vi "HOST_ABEL_Kalman.vi"() -> ()   [LabVIEW 2011]
uses:
  <vilib>/FPGAPlugInAG/PCIe-7852R/niLvFpga_Open_PCIe-7852R.vi
  <vilib>/rvi/interface/common/dynamic/niFpgaDynamicAddResources.vi
  <vilib>/Utility/error.llb/Error Cluster From Error Code.vi
  <vilib>/FPGAPlugInAG/Dynamic/niLvFpga_Run_Dynamic.vi
  <vilib>/RVI Host/nirviSupport.llb/nirviErrorClusterFromErrorCode.vi
  <vilib>/rvi/errors/niLvFpgaAdjustHostInterfaceError.vi
  <vilib>/FPGAPlugInAG/Dynamic/niLvFpga_Reset_Dynamic.vi
  <vilib>/FPGAPlugInAG/Dynamic/niLvFpga_Close_Dynamic.vi
  <vilib>/rvi/interface/nirviOpenFPGA/nirviOpenFPGA.xnode
  FPGA Bitfiles/ABELKalman_FPGATarget_FPGAABELKalman_65AD47D3.lvbitx
  FPGA_ABEL_Kalman.vi
  <vilib>/rvi/interface/nirviMethod/nirviMethod.xnode
  <vilib>/rvi/interface/nirviCloseFPGA/nirviCloseFPGA.xnode
  <vilib>/Analysis/NI_AALBase.lvlib
  <vilib>/rvi/errors/niLvFpgaMergeErrorWithErrorCode.vi
  <vilib>/FPGAPlugInAG/Dynamic/niLvFpga_ConfigureFifo_Dynamic.vi
  <vilib>/FPGAPlugInAG/Dynamic/niLvFpga_StartFifo_Dynamic.vi
  <vilib>/FPGAPlugInAG/Dynamic/niLvFpga_ReadFifo_Dynamic.vi
  <vilib>/FPGAPlugInAG/Dynamic/niLvFpga_WriteFifo_Dynamic.vi
  <vilib>/rvi/interface/nirviMethod/StockFPGA_InlinedMethodWaitForMultipleIRQ.vi
  <vilib>/FPGAPlugInAG/Dynamic/niLvFpga_WaitOnIrq_Dynamic.vi
  <vilib>/FPGAPlugInAG/Dynamic/niLvFpga_AcknowledgeIrq_Dynamic.vi
panel:
  out "Currently Trapped":bool
  out "Number of Trapping Events":u16
  out "Average Time Trapped (ms)":dbl
  in  "Estimate Trap Time":bool
  in  "Threshold (Hz)":dbl=12000.0 min=0.0
  out "Time Recorded (s)":dbl
  in  "Time to Record (s)":dbl=-1.0
  out "Current Modulation Voltages":dbl[][](array[numeric])
  in  "Clear Warnings":bool
  out "y Estimate":dbl
  out "x Estimate":dbl
  in  "Tab Control":enum32{"ABEL Trap Settings"}(tab)
  in  "New Maximum Feedback (V)":dbl=10.0 min=0.0 max=10.0
  out "Current Number of Points per Scan":u8=1
  in  "New Number of Points per Scan":u8=27 min=3 max=32
  in  "New Scan Form":enum8{"Circular", "Square", "Hexagonal"}(ring)=enum."Hexagonal"
  in  "New Spacing (um)":dbl=0.75 min=0.0
  out "Current Scan Form":enum8{"Circular", "Square", "Hexagonal"}(ring)
  out "Current Spacing (um)":dbl
  in  "New Scan Frequency (Hz)":dbl
  out "Current Scan Frequency (Hz)":dbl
  in  "New Radius (um)":dbl min=0.0
  out "Current Radius (um)":dbl
  in  "New Sub-Bin Delay":u16=112
  out "Current Sub-Bin Delay":u16=112
  in  "New Diffusion Constant Estimate (um^2/s)":dbl min=0.0
  out "Current Diffusion Constant Estimate (um^2/s)":dbl
  in  "New Mobility Estimate (um/s/V)":dbl
  out "Current Mobility Estimate (um/s/V)":dbl
  in  "New Beam Waist Estimate (um)":dbl=0.36 min=0.0
  out "Current Beam Waist Estimate (um)":dbl
  in  "New EOD Deflection Scale (um/V)":dbl=0.21 min=0.0
  out "Current EOD Deflection Scale (um/V)":dbl
  out "Current Maximum Feedback (V)":dbl
  out "Current Modulation Frequency (Hz)":dbl
  in  "New Modulation Frequency (Hz)":dbl min=0.0
  out "Current Modulation Radius (um)":dbl
  in  "New Modulation Radius (um)":dbl min=0.0
  in  "New Number of Modulation Points":u8=1 min=1 max=16
  out "Current Number of Modulation Points":u8=1
  in  "New Modulation Angle (degrees)":dbl min=0.0 max=360.0
  out "Current Modulation Angle (degrees)":dbl
  out "On-Chip FIFO Overflow":bool
  in  "Include Mobility Update":bool
  in  "Trap":bool
  out "Feedback DMA Overflow":bool
  out "Feedback":dbl(slide) scale=0.0..1.0
  in  "Update FPGA":bool
  in  "ABEL Stop Button":bool
  out "Ready":bool
  out "Unrecognized Command":bool
  in  "Record":bool
  in  "Top-Level Folder":path=path "C:/Documents and Settings/user/Desktop/Temporary Data"
  out "Position Plot":T1(graph)
  in  "Prefix":string
  out "Mistimed":bool
  out "Recent Photon Count Rate":cluster{dbl[], dbl[]}(graph)
  in  "Update Period (ms)":u32=50 min=1
  in  "Time to Show (s)":dbl=10.0 min=1.0
  out "Photon":dbl(slide) scale=0.0..1.0
  out "Current Voltages":dbl[][](array[numeric])
  out "Photon DMA Overflow":bool
  # "DMA Use"
  # "Scan Parameters"
  # "Beam Parameters"
  # "Trap Parameters"
  # "Modulation Parameters"
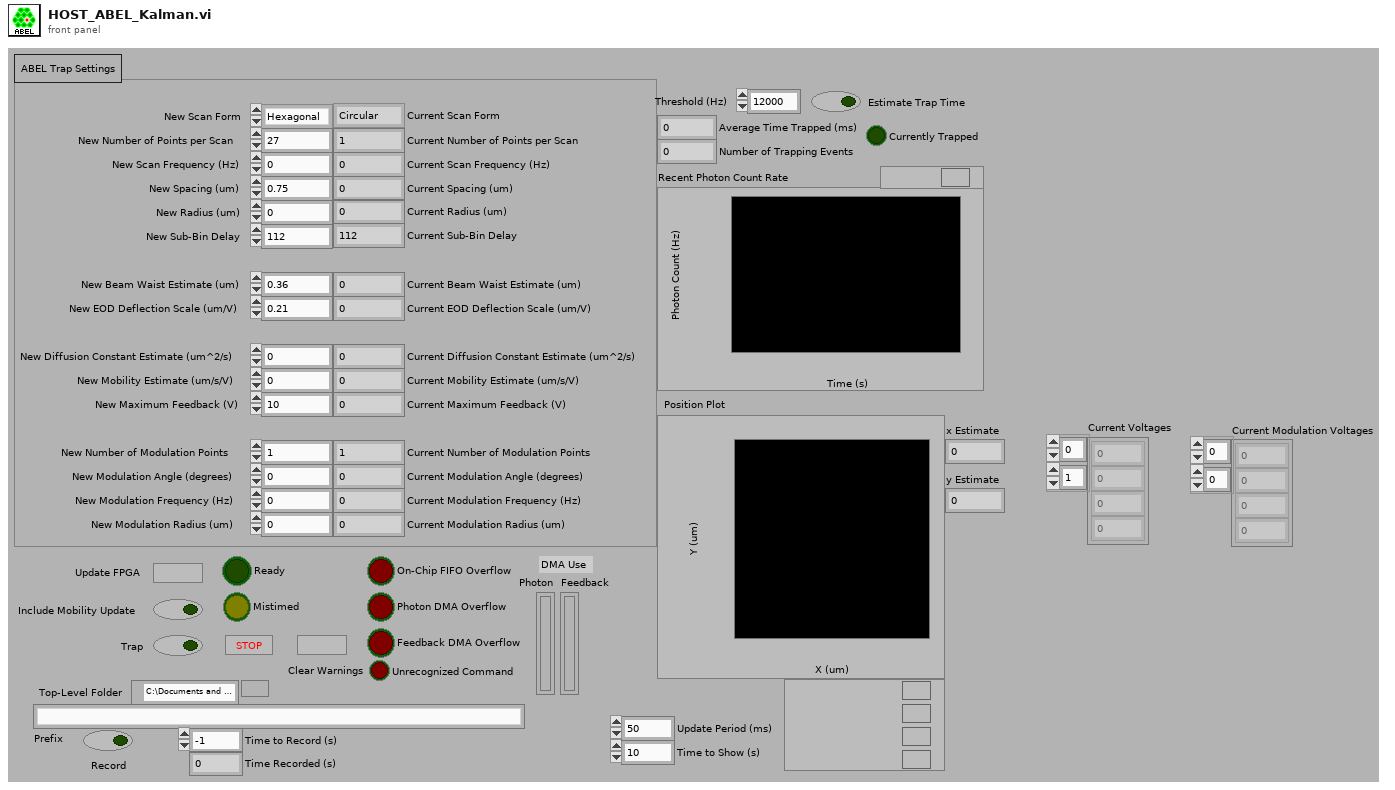
[diagram p1: front panel]
types:
  T1 = cluster{"X coordinates":dbl[], "Y coordinates":dbl[]}[]
  T2 = cluster{"Photon File":refnum<file>, "Feedback File":refnum<file>}
  T3 = enum16{"big-endian, network order", "native, host order", "little-endian"}
  T4 = enum16{"open", "replace", "create", "open or create", "replace or create", "replace or create with confirmation"}
  T5 = cluster{"X coordinates":dbl[], "Y coordinates":dbl[]}
  T6 = cluster{"refnum out":refnum<file>, "refnum out":refnum<file>}
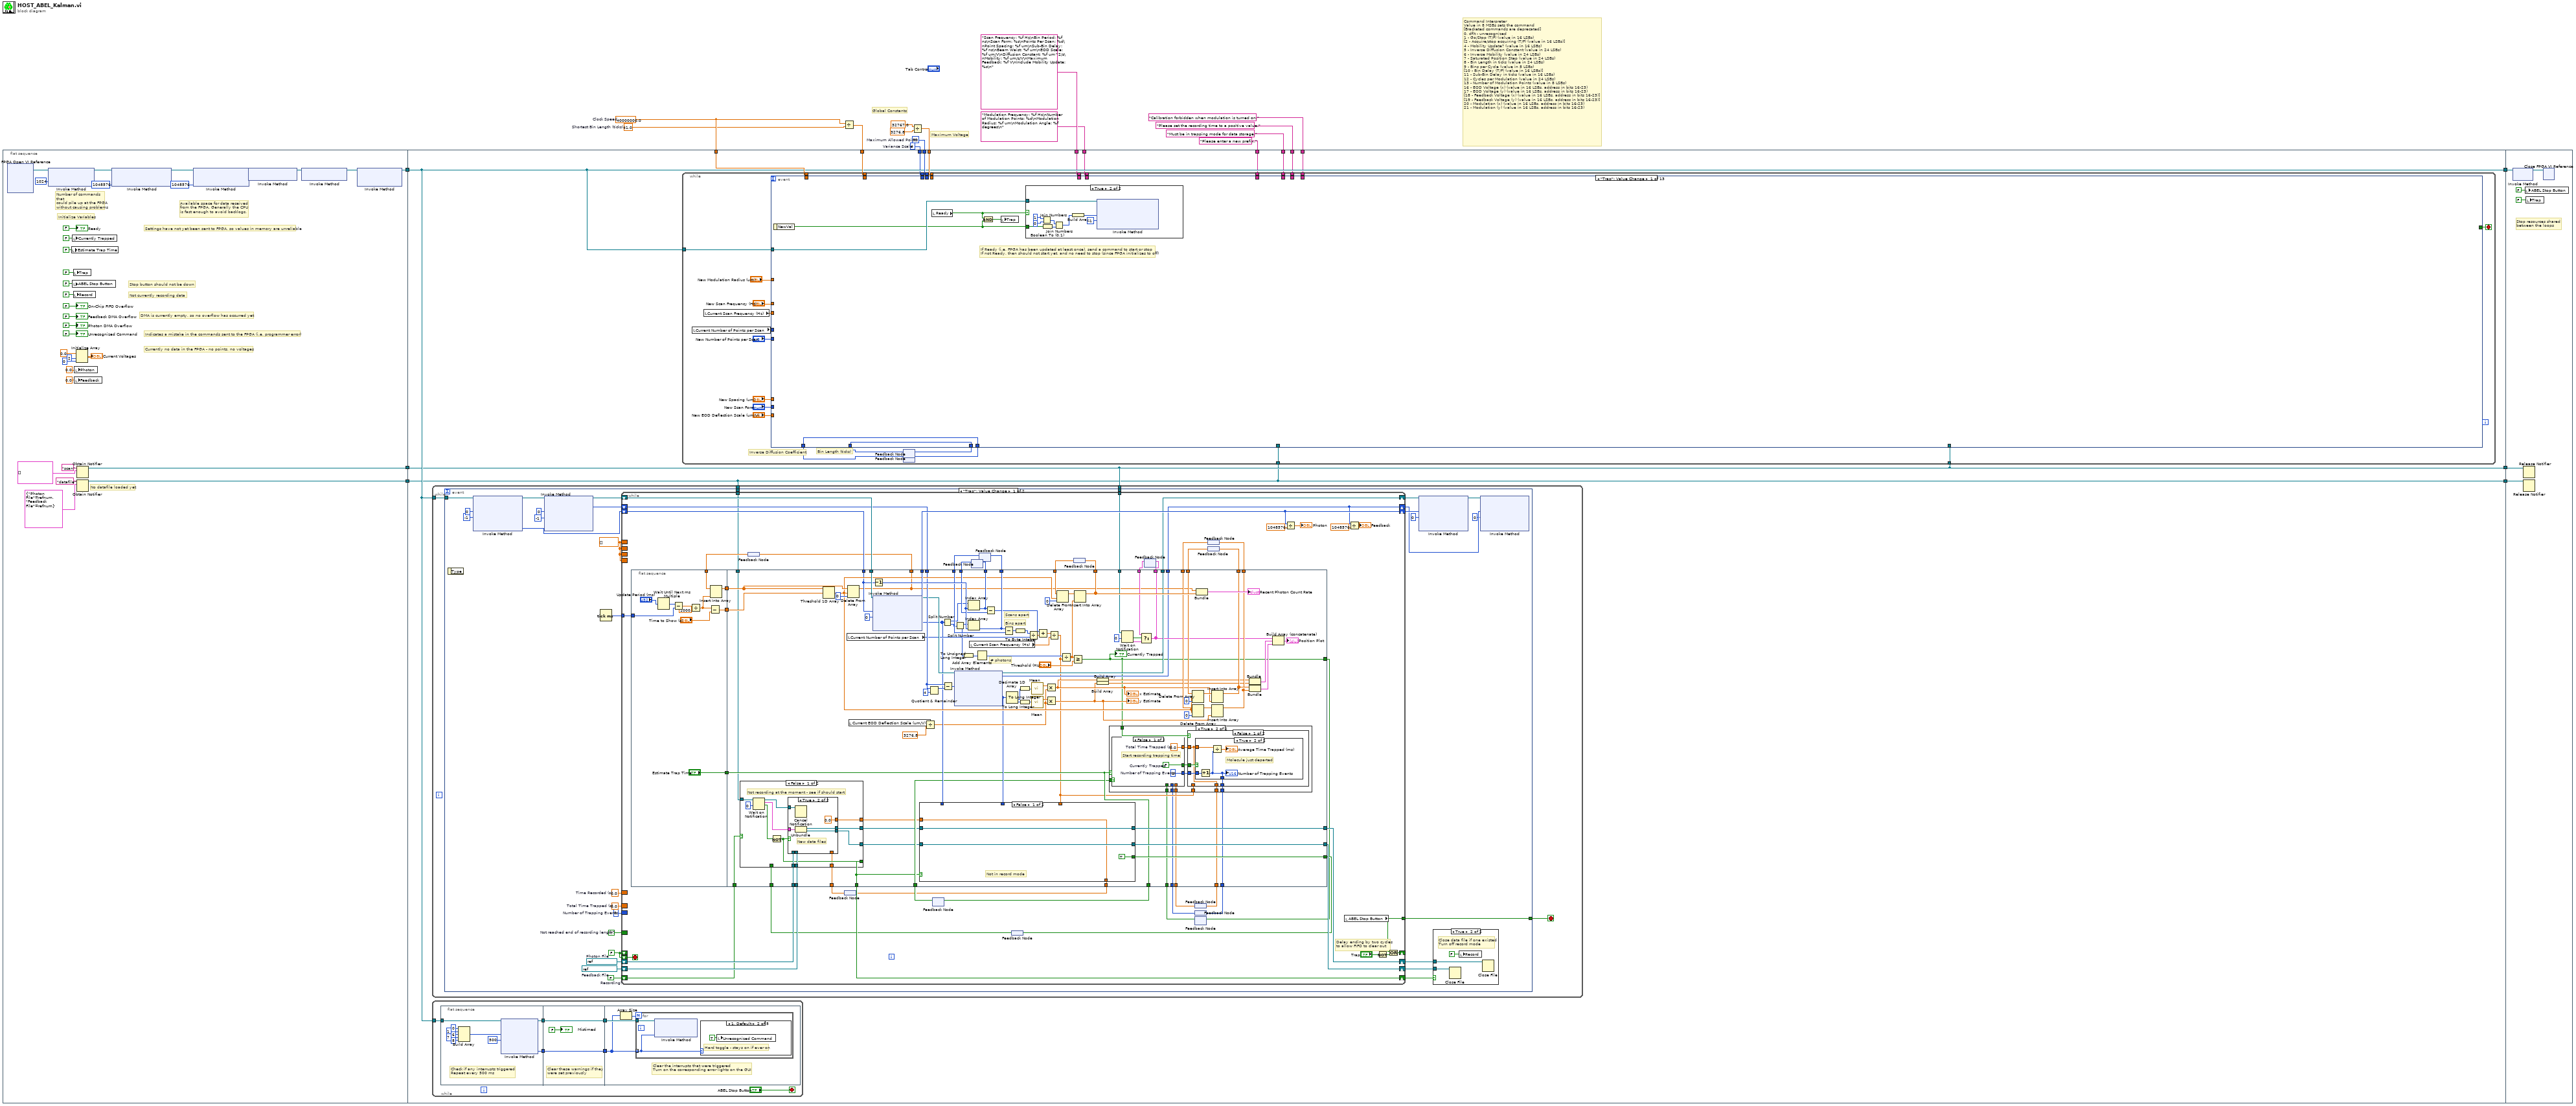
[diagram p0: block diagram]
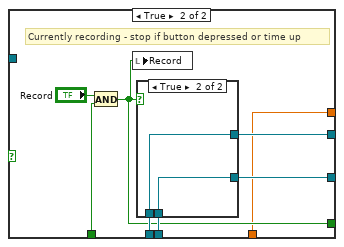
[diagram p4: hidden frame]
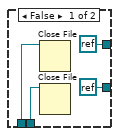
[diagram p5: hidden frame]
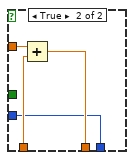
[diagram p8: hidden frame]
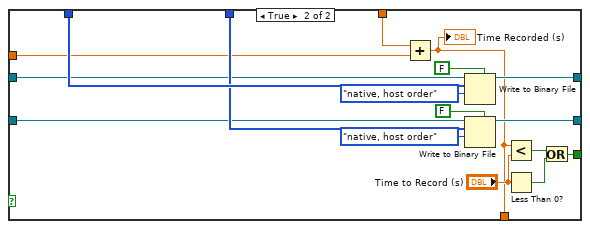
[diagram p10: hidden frame]
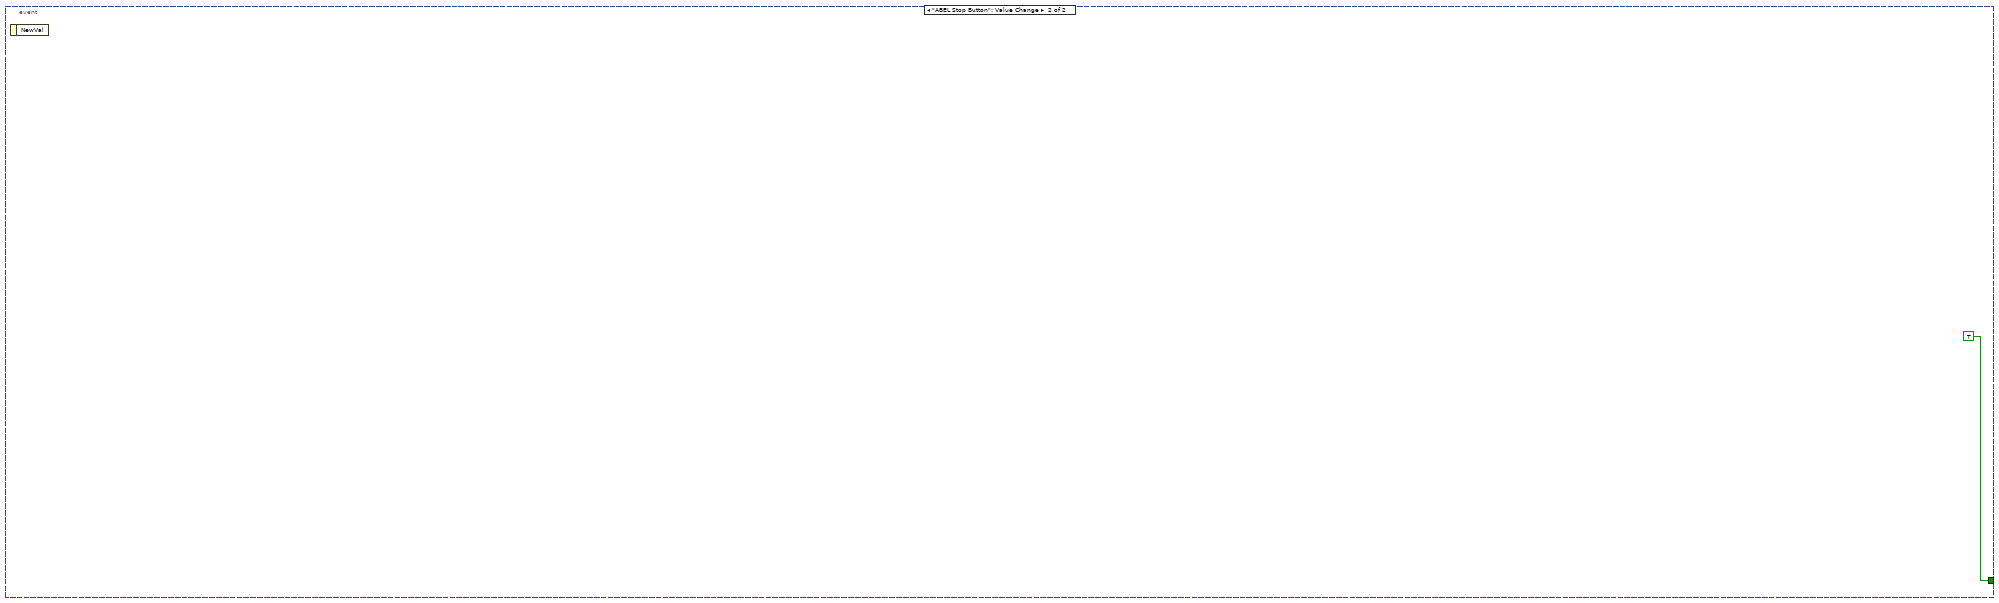
[diagram p11: hidden frame]
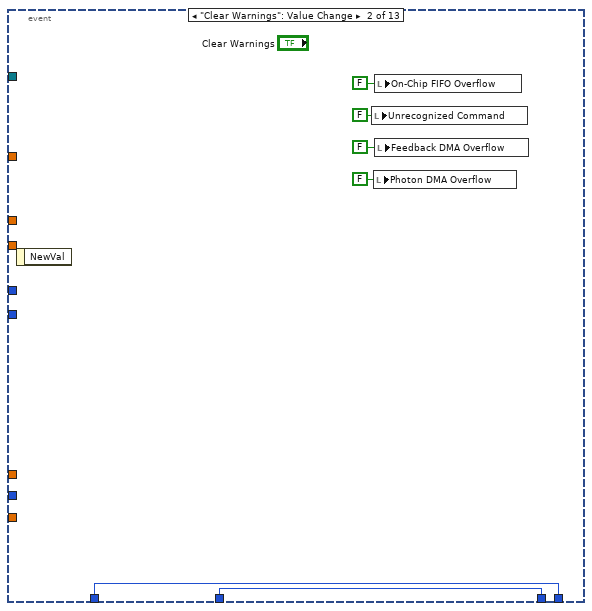
[diagram p13: hidden frame]
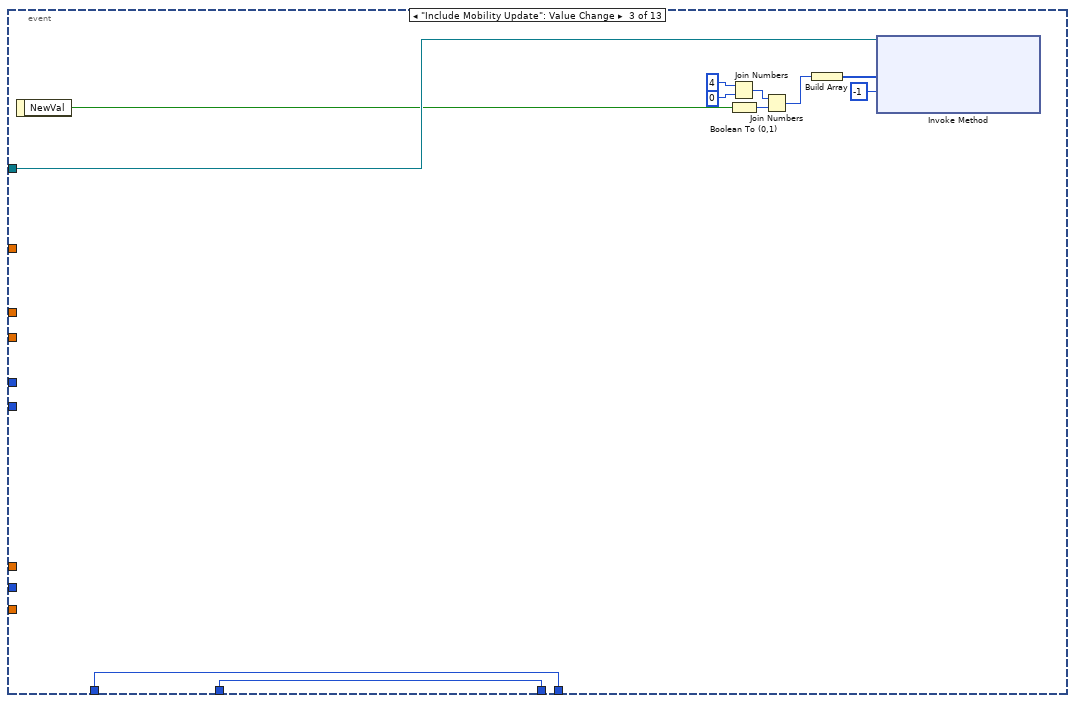
[diagram p14: hidden frame]
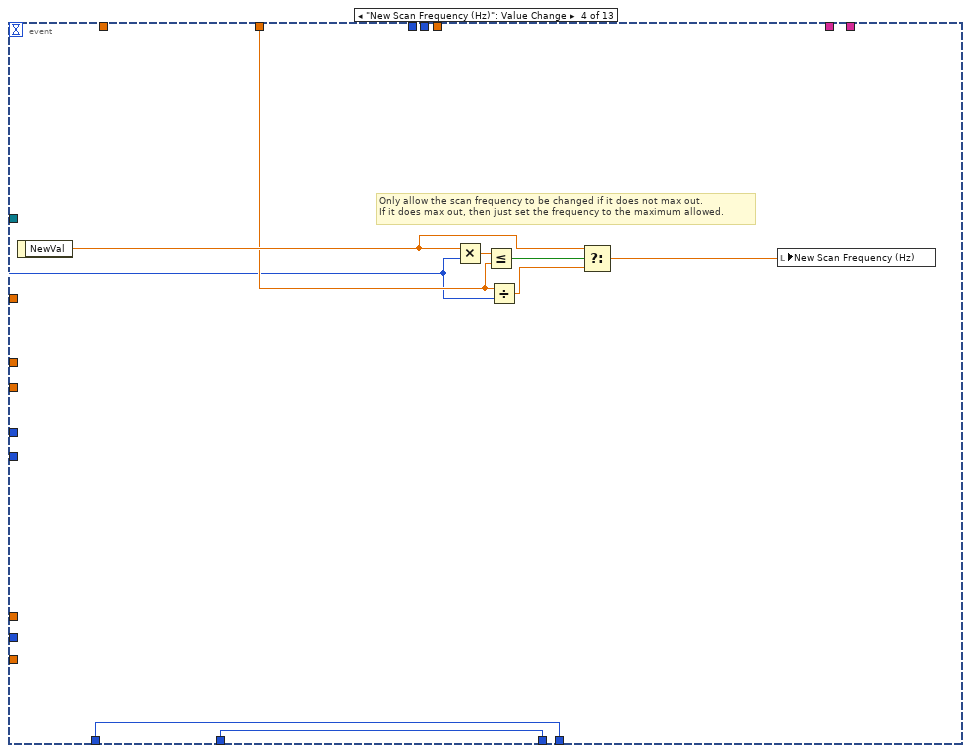
[diagram p15: hidden frame]
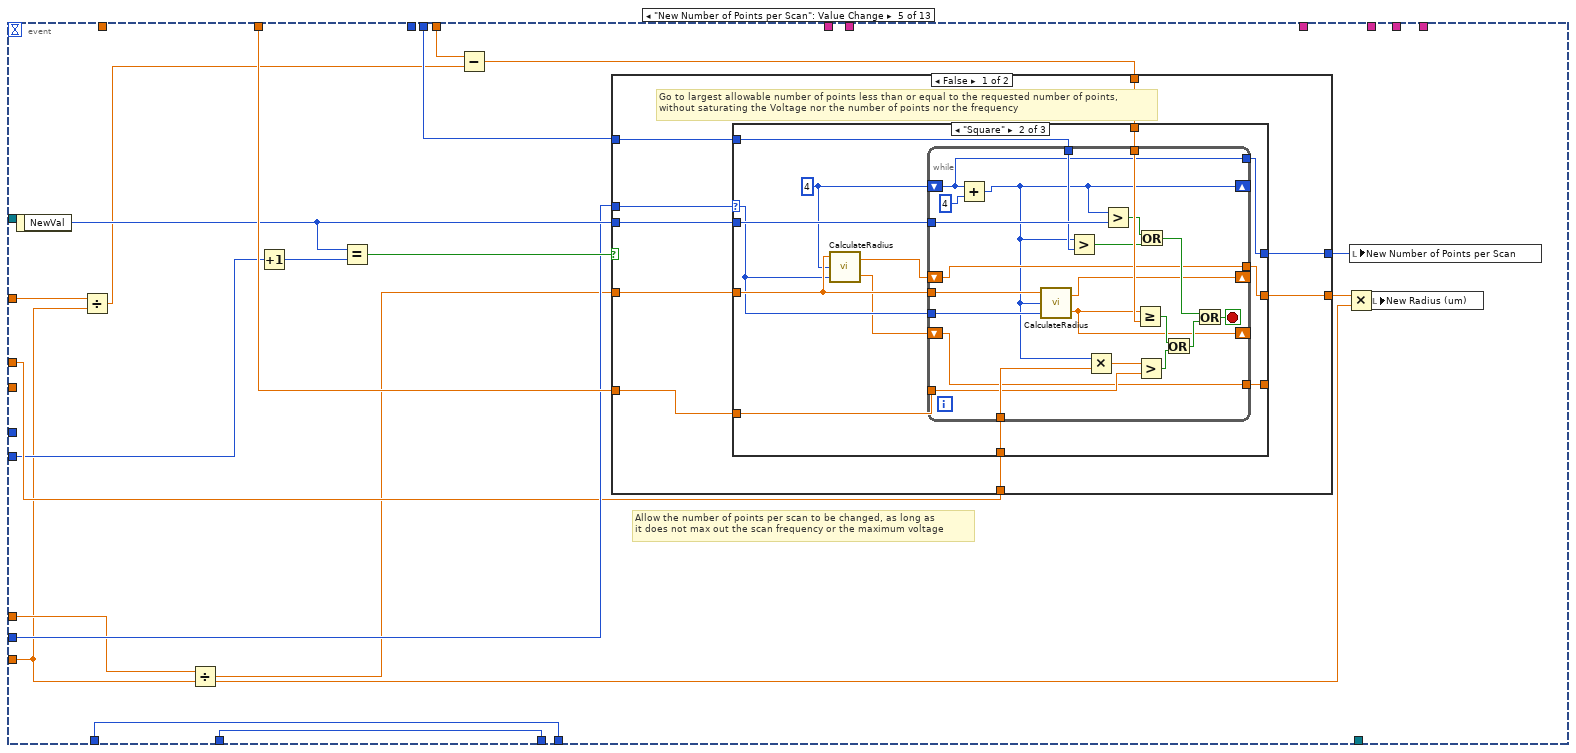
[diagram p16: hidden frame]
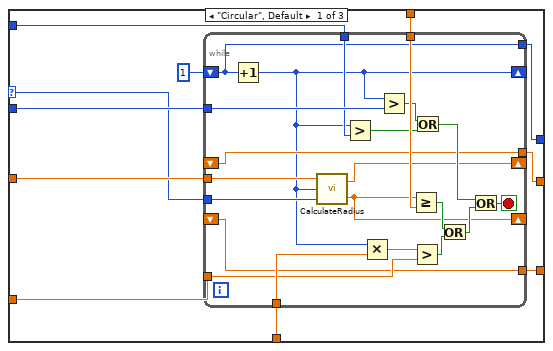
[diagram p17: hidden frame]
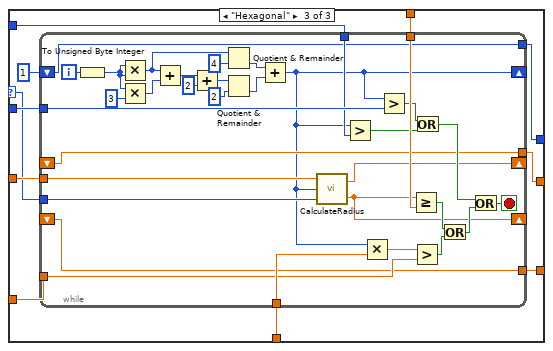
[diagram p18: hidden frame]
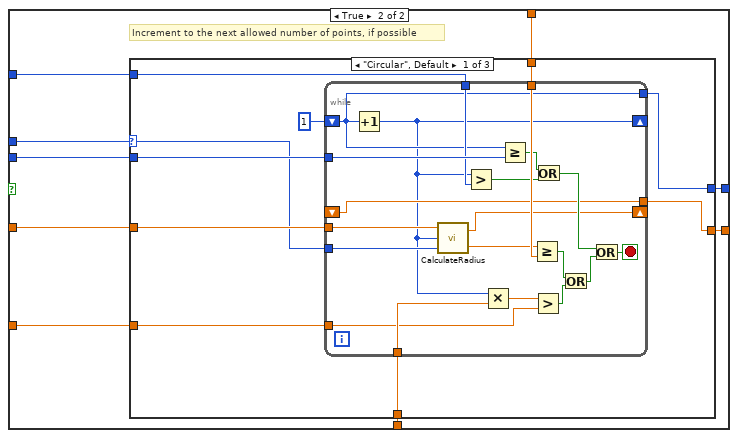
[diagram p19: hidden frame]
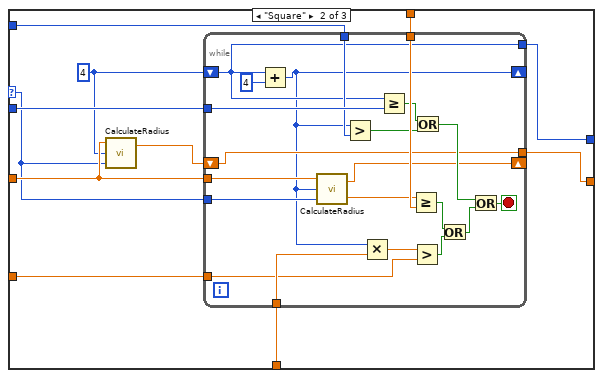
[diagram p20: hidden frame]
diagram:
  w4 = i8 4  # Variance Scale
  w14 = 41.0  # Shortest Bin Length (ticks)
  w16 = 40000000.0  # Clock Speed
  w17 = u8 32  # Maximum Allowed Points
  # "Command Interpreter\nValue in 8 MSBs sets the command\n[Bracketed commands are deprecated]\n0, dflt - unrecognized\n1 - Go/Stop (T/F) (value in 16 LSBs)\n[2 - Acquire/stop acquiring (T/F) (value in 16 LSBs)]\n4 - Mobility Update? (value in 16 LSBs)\n5 - Inverse Diffusion Constant (value in 24 LSBs)\n6 - Inverse Mobility (value in 24 LSBs)\n7 - Saturated Position Step (value in 24 LSBs)\n8 - Bin Length in ticks (value in 24 LSBs)\n9 - Bins per Cycle (value in 8 LSBs)\n[10 - Bin Delay (T/F) (value in 16 LSBs)]\n11 - Sub-Bin Delay in ticks (value in 16 LSBs)\n12 - Cycles per Modulation (value in 24 LSBs)\n13 - Number of Modulation Points (value in 8 LSBs)\n16 - EOD Voltage (x) (value in 16 LSBs, address in bits 16-23)\n17 - EOD Voltage (y) (value in 16 LSBs, address in bits 16-23)\n[18 - Feedback Voltage (x) (value in 16 LSBs, address in bits 16-23)]\n[19 - Feedback Voltage (y) (value in 16 LSBs, address in bits 16-23)]\n20 - Modulation (x) (value in 16 LSBs, address in bits 16-23)\n21 - Modulation (y) (value in 16 LSBs, address in bits 16-23)"
  # "Maximum Voltage"
  # "Global Constants"
  n1 = flat-sequence {
    tunnel: [w36] -> w20
    tunnel: [w40] -> w19
    tunnel: [w33] -> w10
    tunnel: w20 -> [w62]
    tunnel: [w62] -> w18
    tunnel: w17 -> [w66]
    tunnel: w11 -> [w65]
    tunnel: w15 -> [w64]
    tunnel: w16 -> [w63]
    tunnel: w19 -> [w60]
    tunnel: w10 -> [w61]
    tunnel: [w61] -> w9
    tunnel: [w60] -> w8
    tunnel: "Please enter a new prefix." ("message") -> [w59]
    tunnel: "Must be in trapping mode for data storage." ("message") -> [w58]
    tunnel: "Scan Frequency: %f Hz\nBin Period: %f ns\nScan Form: %s\nPoints Per Scan: %d\nPoint Spacing: %f um\nSub-Bin Delay: %f ns\nBeam Waist: %f um\nEOD Scale: %f um/V\nDiffusion Constant: %f um^2/s\nMobility: %f um/s/V\nMaximum Feedback: %f V\nInclude Mobility Update: %s\n" ("format string") -> [w57]
    tunnel: w4 -> [w56]
    tunnel: "Modulation Frequency: %f Hz\nNumber of Modulation Points: %d\nModulation Radius: %f um\nModulation Angle: %f degrees\n" ("format string") -> [w55]
    tunnel: "Calibration forbidden when modulation is turned on." ("message") -> [w54]
    tunnel: "Please set the recording time to a positive value." ("message") -> [w53]
    tunnel: w18 -> [w1258]
    tunnel: w9 -> [w1254]
    tunnel: w8 -> [w1253]
    frame #0 {
      # "No datafile loaded yet"
      # "Available space for data received\nfrom the FPGA. Generally the CPU\nis fast enough to avoid backlogs."
      # "Number of commands that\ncould pile up at the FPGA\nwithout causing problems"
      # "Currently no data in the FPGA - no points, no voltages"
      # "Indicates a mistake in the commands sent to the FPGA (i.e. programmer error)"
      # "DMA is currently empty, so no overflow has occurred yet"
      # "Settings have not yet been sent to FPGA, so values in memory are unreliable"
      # "Not currently recording data"
      # "Stop button should not be down"
      # "Initialize Variables"
      n2 = xnode "FPGA Open VI Reference"() -> ("FPGA VI Reference Out"=w51:refnum<k20>)  [unwired: 2 in, 1 out]
      n3 = xnode "Invoke Method"("FPGA VI Reference In"=w51, "Depth"=u32 1024) -> ("FPGA VI Reference Out"=w49:refnum<k20>)  [unwired: 1 in, 1 out]
      n4 = local write "Estimate Trap Time"(FALSE ("Estimate Trap Time")) -> ()
      n5 = local write "Currently Trapped"(FALSE ("Currently Trapped")) -> ()
      n6 = local write "ABEL Stop Button"(FALSE ("stop")) -> ()
      n7 = local write "Trap"(FALSE ("Trap")) -> ()
      n8 = local write "Record"(FALSE ("Record")) -> ()
      n9 = local write "Photon"(0.0 ("DMA Use")) -> ()
      n10 = local write "Feedback"(0.0 ("DMA Use")) -> ()
      n11 = Initialize Array(0.0 ("element"), 2 ("dimension size"), 0 ("dimension size")) -> (→"Current Voltages":dbl[][])
      n12 = Obtain Notifier(name (unnamed)="scan", notification data type=T1 [] ("appended array")) -> (notifier out=w33:refnum<notifier>)  [unwired: 2 in, 2 out]
      n13 = Obtain Notifier(name (unnamed)="datafile", notification data type=T2 {"Photon File"=refnum, "Feedback File"=refnum}) -> (notifier out=w40:refnum<notifier>)  [unwired: 2 in, 2 out]
      n14 = xnode "Invoke Method"("FPGA VI Reference In"=w49, "Depth"=u32 1048576) -> ("FPGA VI Reference Out"=w37:refnum<k20>)  [unwired: 1 in, 1 out]
      n15 = xnode "Invoke Method"("FPGA VI Reference In"=w37, "Depth"=u32 1048576) -> ("FPGA VI Reference Out"=w26:refnum<k20>)  [unwired: 1 in, 1 out]
      n16 = xnode "Invoke Method"("FPGA VI Reference In"=w26) -> ("FPGA VI Reference Out"=w25:refnum<k20>)  [unwired: 1 in, 1 out]
      n17 = xnode "Invoke Method"("FPGA VI Reference In"=w25) -> ("FPGA VI Reference Out"=w24:refnum<k20>)  [unwired: 1 in, 1 out]
      n18 = xnode "Invoke Method"("FPGA VI Reference In"=w24) -> ("FPGA VI Reference Out"=w36:refnum<k20>)  [unwired: 2 in, 1 out]
      "Ready" <- FALSE ("Ready")
      "Unrecognized Command" <- FALSE ("Incorrect Command")
      "Photon DMA Overflow" <- FALSE ("Overflow")
      "Feedback DMA Overflow" <- FALSE ("Feedback DMA Overflow")
      "On-Chip FIFO Overflow" <- FALSE ("On-Chip FIFO Overflow")
    }
    frame #1 {
      n19 = while {
        tunnel: w60 -> [w70]
        tunnel: w62 -> [w69]
        tunnel: w61 -> [w68]
        stop <- w67 stop-if-true
        n20 = event shown="[0] \"Trap\": Value Change" {
          selector: _ -> [_ _]
          dyn-events: _ -> [_ _]
          timeout: _ -> [_ _]
          tunnel: w70 -> [w101 _]
          tunnel: w69 -> [w83 _]
          tunnel: w68 -> [w93 _]
          tunnel: [w88 TRUE ("ABEL Stop Button")] -> w67
          event "Trap": Value Change {
            w72 = u16 0  # Number of Trapping Events
            w71 = 0.0  # Total Time Trapped (s)
            w73 = 0.0  # Time Recorded (s)
            w74 = dbl[] []
            w84 = TRUE  # Not reached end of recording length?
            w87 = FALSE
            w86 = refnum<k0> refnum  # Feedback File
            w99 = refnum<k0> refnum  # Photon File
            w100 = FALSE  # Recording?
            n21 = event-data() -> ()  [unwired: 1 in, 1 out]
            n22 = xnode "Invoke Method"("FPGA VI Reference In"=w83, "Number of Elements"=u32 0, "Timeout (ms)"=-1) -> ("FPGA VI Reference Out"=w82:refnum<k20>, "Elements Remaining"=w78:u32)  [unwired: 1 in, 2 out]
            n23 = xnode "Invoke Method"("FPGA VI Reference In"=w82, "Number of Elements"=u32 0, "Timeout (ms)"=-1) -> ("FPGA VI Reference Out"=w81:refnum<k20>, "Elements Remaining"=w77:u32)  [unwired: 1 in, 2 out]
            n24 = Tick Count (ms)() -> (millisecond timer value=w96:u32)
            n25 = while {
              shift-right: [w136] -> w94
              shift-left: w78 -> [w156]
              shift-right: [w151] -> w97
              shift-left: w99 -> [w150]
              tunnel: w101 -> [w114]
              shift-right: [w149] -> w98
              shift-left: w100 -> [w115]
              tunnel: w96 -> [w143]
              shift-right: [w130] -> w90
              shift-left: w77 -> [w135]
              tunnel: w93 -> [w133]
              shift-right: [w129] -> w92
              shift-left: w81 -> [w157]
              tunnel: [w126] -> w88
              shift-right: [w125] -> _
              shift-left: w87 -> [_]
              shift-left: w87 -> [w124]
              shift-right: [w122] -> w85
              shift-left: w86 -> [w123]
              border: w74 -> [_]
              border: w74 -> [_]
              border: w74 -> [_]
              border: w74 -> [_]
              border: w84 -> [_]
              border: w73 -> [_]
              border: w71 -> [_]
              border: w72 -> [_]
              stop <- w124 stop-if-true
              # "Delay ending by two cycles\nto allow FIFO to clear out"
              n26 = flat-sequence {
                tunnel: w146 -> [w167]
                tunnel: [w166] -> w145
                tunnel: [w162] -> w144
                tunnel: w143 -> [w159]
                tunnel: ["Estimate Trap Time"] -> w118
                tunnel: w157 -> [w264]
                tunnel: w156 -> [w222]
                tunnel: [w263] -> w136
                tunnel: [w258] -> w155
                tunnel: [w257] -> w154
                tunnel: w153 -> [w256]
                tunnel: w152 -> [w255]
                tunnel: [w251] -> w151
                tunnel: w150 -> [w175]
                tunnel: w115 -> [w177]
                tunnel: [w171] -> w149
                tunnel: w145 -> [w249]
                tunnel: w144 -> [w250]
                tunnel: w142 -> [w247]
                tunnel: [w187] -> w141
                tunnel: [w243] -> w140
                tunnel: w139 -> [w239]
                tunnel: w138 -> [w238]
                tunnel: [w221] -> w137
                tunnel: w135 -> [w228]
                tunnel: [w186] -> w130
                tunnel: [w220] -> w134
                tunnel: w133 -> [w218]
                tunnel: [w211] -> w129
                tunnel: w123 -> [w176]
                tunnel: [w203] -> w122
                tunnel: [w197] -> w121
                tunnel: w120 -> [w196]
                tunnel: [w193] -> w111
                tunnel: w112 -> [w170]
                tunnel: [w192] -> w119
                tunnel: w118 -> [w191]
                tunnel: [w191] -> w117
                tunnel: w116 -> [w190]
                tunnel: [w184] -> w109
                tunnel: w110 -> [w183]
                tunnel: [w182] -> w108
                tunnel: w107 -> [w181]
                tunnel: [w180] -> w105
                tunnel: w106 -> [w179]
                tunnel: w114 -> [w178]
                tunnel: w113 -> [w174]
                frame #0 {
                  n27 = Wait Until Next ms Multiple(millisecond multiple="Update Period (ms)") -> (millisecond timer value=w160:u32)
                  n28 = Subtract(x=w160, y=w159) -> (x-y=w161:u32)
                  n29 = Divide(x=w161, y=1000.0) -> (x/y=w164:dbl)
                  n30 = Subtract(x=w164, y="Time to Show (s)") -> (x-y=w162:dbl)
                  n31 = Insert Into Array(array=w167, new element=w164) -> (w166:dbl[])  [unwired: 1 in]
                }
                frame #1 {
                  # "Scans apart"
                  # "Bins apart"
                  # "# photons"
                  n32 = case shown="False" w177 {
                    tunnel: w178 -> [w275 _]
                    tunnel: w176 -> [w273 w290]
                    tunnel: w175 -> [w272 w289]
                    tunnel: w174 -> [_ w291]
                    tunnel: [w270 w288] -> w173
                    tunnel: [w271 w287] -> w172
                    tunnel: [w268 w286] -> w171
                    tunnel: w170 -> [w267 w285]
                    tunnel: [w266 w285] -> w169
                    frame False {
                      # "Not recording at the moment - see if should start"
                      n33 = Wait on Notification(notifier=w275, timeout in ms (-1)=0) -> (notifier out=w265:refnum<notifier>, notification=w274:T2, timed out?=w269:bool)  [unwired: 2 in, 1 out]
                      n34 = Not(x=w269) -> (.not. x?=w268:bool)
                      n35 = case shown="True" w268 {
                        tunnel: w274 -> [_ w284]
                        tunnel: [w278 w283] -> w270
                        tunnel: [w279 w282] -> w271
                        tunnel: w273 -> [w279 _]
                        tunnel: w272 -> [w278 _]
                        tunnel: [w277 0.0] -> w266
                        tunnel: w267 -> [w277 _]
                        tunnel: w265 -> [_ w280]
                        frame False {
                        }
                        frame True {
                          # "New data files"
                          n36 = Cancel Notification(0:w280) -> ()  [unwired: 1 in, 3 out]
                          n37 = Unbundle(w284) -> ("Photon File"=w283:refnum<file>, "Feedback File"=w282:refnum<file>)
                        }
                      }
                    }
                    frame True {
                      # "Currently recording - stop if button depressed or time up"
                      n38 = And(x="Record", y=w291) -> (x .and. y?=w286:bool)
                      n39 = local write "Record"(w286) -> ()
                      n40 = case shown="True" w286 {
                        tunnel: w290 -> [w296 w298]
                        tunnel: w289 -> [w295 w297]
                        tunnel: [refnum<k0> refnum w297] -> w288
                        tunnel: [refnum<k0> refnum w298] -> w287
                        frame False {
                          n41 = Close File(refnum=w295) -> ()  [unwired: 1 in, 2 out]
                          n42 = Close File(refnum=w296) -> ()  [unwired: 1 in, 2 out]
                        }
                        frame True {
                        }
                      }
                    }
                  }
                  n43 = Threshold 1D Array(2:w250, 3:w249) -> (0:w240:dbl)  [unwired: 1 in]
                  n44 = local read "Current Number of Points per Scan"() -> (w224:u8)
                  n45 = Delete From Array(array=w249, length=w240, index=0) -> (array with subset deleted=w187:dbl[])  [unwired: 1 out]
                  n46 = local read "Current EOD Deflection Scale (um/V)"() -> (w205:dbl)
                  n47 = xnode "Invoke Method"("FPGA VI Reference In"=w264, "Number of Elements"=w222, "Timeout (ms)"=0) -> ("FPGA VI Reference Out"=w227:refnum<k20>, "Data"=w212:u32[], "Elements Remaining"=w263:u32)  [unwired: 1 in, 1 out]
                  n48 = Decrement(x=w222) -> (x-1=w261:u32)
                  n49 = Divide(x=w205, y=3276.8) -> (x/y=w204:dbl)
                  n50 = Quotient & Remainder(x=w228, y=u32 4) -> (x-y*floor(x/y)=w229:u32)  [unwired: 1 out]
                  n51 = Split Number(x=w212) -> (hi(x)=w233:u16[], lo(x)=w234:u16[])
                  n52 = Subtract(x=w228, y=w229) -> (x-y=w226:u32)
                  n53 = xnode "Invoke Method"("FPGA VI Reference In"=w227, "Number of Elements"=w226) -> ("FPGA VI Reference Out"=w211:refnum<k20>, "Data"=w202:u32[], "Elements Remaining"=w186:u32)  [unwired: 2 in, 1 out]
                  n54 = Split Number(x=w234) -> (hi(x)=w232:u8[], lo(x)=w231:u8[])
                  n55 = To Unsigned Long Integer(number=w231) -> (unsigned 32bit integer=w262:u32[])
                  n56 = Index Array(array=w233, index=w261) -> (element=w258:u16)
                  n57 = Index Array(array=w232, index=w261) -> (element=w257:u8)
                  n58 = local read "Current Scan Frequency (Hz)"() -> (w195:dbl)
                  n59 = Add Array Elements(numeric array=w262) -> (sum=w194:u32)
                  n60 = Subtract(x=w258, y=w256) -> (x-y=w252:u16)
                  n61 = Subtract(x=w257, y=w255) -> (x-y=w254:u8)
                  n62 = Decimate 1D Array(w202) -> (w210:u32[], w208:u32[])  [unwired: 2 out]
                  n63 = To Byte Integer(number=w254) -> (8bit integer=w253:i8)
                  n64 = To Long Integer(number=w210) -> (32bit integer=w209:i32[])
                  n65 = To Long Integer(number=w208) -> (32bit integer=w207:i32[])
                  n66 = Divide(x=w253, y=w224) -> (x/y=w260:dbl)
                  n67 = call <vilib>:"Mean.vi"("X"=w209) -> ("mean"=w225:dbl)  [unwired: 1 out]
                  n68 = call <vilib>:"Mean.vi"("X"=w207) -> ("mean"=w223:dbl)  [unwired: 1 out]
                  n69 = Add(x=w252, y=w260) -> (x+y=w259:dbl)
                  n70 = Multiply(x=w225, y=w204) -> (x*y=w201:dbl)
                  "x Estimate" <- w201
                  n71 = Multiply(x=w223, y=w204) -> (x*y=w200:dbl)
                  "y Estimate" <- w200
                  n72 = Divide(x=w259, y=w195) -> (x/y=w185:dbl)
                  n73 = case shown="False" w171 {
                    tunnel: [w334 w351] -> w251
                    tunnel: w173 -> [w334 w337]
                    tunnel: w212 -> [_ w348]
                    tunnel: w172 -> [w333 w336]
                    tunnel: [w333 w345] -> w203
                    tunnel: w202 -> [_ w344]
                    tunnel: w185 -> [_ w339]
                    tunnel: [w332 w338] -> w193
                    tunnel: w169 -> [w332 w335]
                    tunnel: [TRUE w340] -> w192
                    frame False {
                      # "Not in record mode"
                    }
                    frame True {
                      n74 = Add(x=w339, y=w335) -> (x+y=w338:dbl)
                      "Time Recorded (s)" <- w338
                      n75 = Write to Binary File(file (use dialog)=w337, data=w348, 5:FALSE ("prepend array or string size? (T)"), 9:T3."native, host order" ("byte order (0:big-endian, network order)")) -> (refnum out=w351:refnum<file>)  [unwired: 2 in, 2 out]
                      n76 = Write to Binary File(file (use dialog)=w336, data=w344, 5:FALSE ("prepend array or string size? (T)"), 9:T3."native, host order" ("byte order (0:big-endian, network order)")) -> (refnum out=w345:refnum<file>)  [unwired: 2 in, 2 out]
                      n77 = Less?(x=w338, y="Time to Record (s)") -> (x < y?=w342:bool)
                      n78 = Less Than 0?(x="Time to Record (s)") -> (x < 0?=w341:bool)
                      n79 = Or(x=w342, y=w341) -> (x .or. y?=w340:bool)
                    }
                  }
                  n80 = Delete From Array(array=w247, length=w240, index=0) -> (array with subset deleted=w244:dbl[])  [unwired: 1 out]
                  n81 = Divide(x=w194, y=w185) -> (x/y=w189:dbl)
                  n82 = Greater Or Equal?(x=w189, y="Threshold (Hz)") -> (x >= y?=w180:bool)
                  "Currently Trapped" <- w180
                  n83 = Insert Into Array(array=w244, new element=w189) -> (w243:dbl[])  [unwired: 1 in]
                  n84 = Build Array(w201) -> (w215:dbl[])
                  n85 = Build Array(w200) -> (w214:dbl[])
                  n86 = case shown="True" w191 {
                    tunnel: w190 -> [_ w311]
                    tunnel: w180 -> [_ w310]
                    tunnel: w185 -> [_ w308]
                    tunnel: [w300 w305] -> w182
                    tunnel: [w299 w304] -> w184
                    tunnel: w183 -> [w299 w303]
                    tunnel: w181 -> [w300 w302]
                    tunnel: w179 -> [_ w301]
                    frame False {
                      # "Not recording trapping time"
                    }
                    frame True {
                      n87 = case shown="False" w311 {
                        tunnel: [w327 w329] -> w309
                        tunnel: [w326 w328] -> w307
                        tunnel: [w325 w330] -> w306
                        tunnel: w303 -> [_ w330]
                        tunnel: w302 -> [_ w329]
                        tunnel: w301 -> [_ w328]
                        frame False {
                          w325 = u16 0  # Number of Trapping Events
                          w326 = FALSE  # Currently Trapped
                          w327 = 0.0  # Total Time Trapped (s)
                          # "Start recording trapping time"
                        }
                        frame True {
                          # "Continue recording\ntrapping time"
                        }
                      }
                      n88 = case shown="False" w310 {
                        tunnel: w309 -> [w313 w324]
                        tunnel: w308 -> [_ w323]
                        tunnel: w307 -> [w315 _]
                        tunnel: w306 -> [w314 w321]
                        tunnel: [w313 w322] -> w305
                        tunnel: [w312 w321] -> w304
                        frame False {
                          n89 = case shown="True" w315 {
                            tunnel: w314 -> [w316 w320]
                            tunnel: w313 -> [_ w319]
                            tunnel: [w316 w317] -> w312
                            frame False {
                            }
                            frame True {
                              # "Molecule just departed"
                              n90 = Increment(x=w320) -> (x+1=w317:u16)
                              "Number of Trapping Events" <- w317
                              n91 = Divide(x=w319, y=w317) -> (x/y=→"Average Time Trapped (ms)":dbl)
                            }
                          }
                        }
                        frame True {
                          n92 = Add(x=w324, y=w323) -> (x+y=w322:dbl)
                        }
                      }
                    }
                  }
                  n93 = Wait on Notification(notifier=w218, timeout in ms (-1)=0) -> (notification=w198:T1, timed out?=w199:bool)  [unwired: 2 in, 2 out]
                  n94 = Select(t=w196, s=w199, f=w198) -> (s? t:f=w197:T1)
                  n95 = Delete From Array(array=w239, length=w240, index=0) -> (array with subset deleted=w237:dbl[])  [unwired: 1 out]
                  n96 = Delete From Array(array=w238, length=w240, index=0) -> (array with subset deleted=w236:dbl[])  [unwired: 1 out]
                  n97 = Bundle(w187, w243) -> (→"Recent Photon Count Rate":cluster{dbl[], dbl[]})  [unwired: 1 in]
                  n98 = Insert Into Array(array=w237, new element=w201) -> (w221:dbl[])  [unwired: 1 in]
                  n99 = Insert Into Array(array=w236, new element=w200) -> (w220:dbl[])  [unwired: 1 in]
                  n100 = Bundle(w215, w214) -> (w216:cluster{dbl[], dbl[]})  [unwired: 1 in]
                  n101 = Bundle(w221, w220) -> (w217:cluster{dbl[], dbl[]})  [unwired: 1 in]
                  n102 = Build Array (concatenate)(w197, w216, w217) -> (→"Position Plot":T1)
                }
              }
              n103 = feedback-in #1(w141) -> ()
              n104 = feedback #1() -> (w146:dbl[])
              n105 = feedback-in #2(w111) -> ()
              n106 = feedback #2() -> (w112:dbl)
              n107 = feedback-in #3(w117) -> ()
              n108 = feedback #3() -> (w116:bool)  [unwired: 1 in]
              n109 = feedback-in #4(w155) -> ()
              n110 = feedback #4() -> (w153:u16)  [unwired: 1 in]
              n111 = feedback-in #5(w154) -> ()
              n112 = feedback #5() -> (w152:u8)  [unwired: 1 in]
              n113 = feedback-in #6(w119) -> ()
              n114 = feedback #6() -> (w113:bool)
              n115 = feedback-in #7(w140) -> ()
              n116 = feedback #7() -> (w142:dbl[])
              n117 = feedback-in #8(w121) -> ()
              n118 = feedback #8() -> (w120:T1)  [unwired: 1 in]
              n119 = feedback-in #9(w108) -> ()
              n120 = feedback #9() -> (w107:dbl)
              n121 = feedback-in #10(w109) -> ()
              n122 = feedback #10() -> (w110:u16)
              n123 = feedback-in #11(w105) -> ()
              n124 = feedback #11() -> (w106:bool)  [unwired: 1 in]
              n125 = feedback-in #12(w134) -> ()
              n126 = feedback #12() -> (w138:dbl[])
              n127 = feedback-in #13(w137) -> ()
              n128 = feedback #13() -> (w139:dbl[])
              n129 = Divide(x=w136, y=1048576.0 ("Depth")) -> (x/y=→"Photon":dbl)
              n130 = local read "ABEL Stop Button"() -> (w126:bool)
              n131 = Divide(x=w130, y=1048576.0 ("Depth")) -> (x/y=→"Feedback":dbl)
              n132 = Not(x="Trap") -> (.not. x?=w128:bool)
              n133 = Or(x=w126, y=w128) -> (x .or. y?=w125:bool)
            }
            n134 = xnode "Invoke Method"("FPGA VI Reference In"=w92, "Number of Elements"=w94, "Timeout (ms)"=0) -> ("FPGA VI Reference Out"=w91:refnum<k20>)  [unwired: 1 in, 3 out]
            n135 = case shown="True" w98 {
              tunnel: w97 -> [_ w104]
              tunnel: w85 -> [_ w102]
              frame False {
              }
              frame True {
                # "Close data file if one existed\nTurn off record mode"
                n136 = Close File(refnum=w102) -> ()  [unwired: 1 in, 2 out]
                n137 = local write "Record"(FALSE ("Record")) -> ()
                n138 = Close File(refnum=w104) -> ()  [unwired: 1 in, 2 out]
              }
            }
            n139 = xnode "Invoke Method"("FPGA VI Reference In"=w91, "Number of Elements"=w90, "Timeout (ms)"=0) -> ()  [unwired: 1 in, 4 out]
          }
          event "ABEL Stop Button": Value Change {
            n140 = event-data() -> ()  [unwired: 1 in, 1 out]
          }
        }
      }
      n141 = while {
        tunnel: w62 -> [w1229]
        stop <- "ABEL Stop Button" stop-if-true
        n142 = flat-sequence {
          tunnel: w1229 -> [w1239]
          tunnel: [w1236] -> w1228
          tunnel: [w1235] -> w1226
          tunnel: w1228 -> [w1242]
          tunnel: [w1242] -> w1227
          tunnel: w1226 -> [w1241]
          tunnel: [w1241] -> w1225
          tunnel: w1227 -> [w1243]
          tunnel: w1225 -> [w1244]
          frame #0 {
            # "Check if any interrupts triggered\nRepeat every 500 ms"
            n143 = Build Array(0 ("element"), 1 ("element"), 6 ("element"), 7 ("element"), 8 ("element")) -> (w1237:i32[])
            n144 = xnode "Invoke Method"("FPGA VI Reference In"=w1239, "IRQ Number(s)"=w1237, "Timeout (ms)"=500) -> ("FPGA VI Reference Out"=w1235:refnum<k20>, "IRQ(s) Asserted"=w1236:i32[])  [unwired: 1 in, 2 out]
          }
          frame #1 {
            # "Clear these warnings if they\nwere set previously"
            "Mistimed" <- FALSE ("Mistimed")
          }
          frame #2 {
            # "Clear the interrupts that were triggered\nTurn on the corresponding error lights on the GUI"
            n145 = Array Size(array=w1243) -> (size(s)=w1245:i32)
            n146 = for {
              N: w1245 -> [_]
              tunnel: w1244 -> [w1247]
              tunnel: w1243 -> [w1246] mode=indexing
              n147 = xnode "Invoke Method"("FPGA VI Reference In"=w1247, "IRQ Number(s)"=w1246) -> ()  [unwired: 1 in, 2 out]
              n148 = case shown="1, Default" w1246 {
                frame 0 {
                  # "Soft toggle - cleared after 0.5 s"
                  n149 = local write "Mistimed"(TRUE ("Overflow")) -> ()
                }
                frame 1, Default {
                  # "Hard toggle - stays on if ever on"
                  n150 = local write "Unrecognized Command"(TRUE ("Incorrect Command")) -> ()
                }
                frame 6 {
                  # "Hard toggle - stays on if ever on"
                  n151 = local write "On-Chip FIFO Overflow"(TRUE ("Mistimed")) -> ()
                }
                frame 7 {
                  # "Hard toggle - stays on if ever on"
                  n152 = local write "Photon DMA Overflow"(TRUE ("Mistimed")) -> ()
                }
                frame 8 {
                  # "Hard toggle - stays on if ever on"
                  n153 = local write "Feedback DMA Overflow"(TRUE ("Mistimed")) -> ()
                }
              }
            }
          }
        }
      }
      n154 = while {
        tunnel: w62 -> [w378]
        tunnel: w66 -> [w377]
        tunnel: w65 -> [w376]
        tunnel: w64 -> [w375]
        tunnel: w63 -> [w374]
        tunnel: w60 -> [w368]
        tunnel: w61 -> [w366]
        tunnel: w59 -> [w360]
        tunnel: w58 -> [w359]
        tunnel: w57 -> [w358]
        tunnel: w56 -> [w357]
        tunnel: w55 -> [w355]
        tunnel: w54 -> [w354]
        tunnel: w53 -> [w353]
        stop <- w379 stop-if-true
        # "Inverse Diffusion Coefficient"
        # "Bin Length (ticks)"
        n155 = local read "Current Number of Points per Scan"() -> (w369:u8)
        n156 = local read "Current Scan Frequency (Hz)"() -> (w365:dbl)
        n157 = feedback #14() -> (w363:u16)  [unwired: 1 in]
        n158 = feedback #15() -> (w361:u32)  [unwired: 1 in]
        n159 = event shown="[0] \"Trap\": Value Change" {
          selector: _ -> [_ _ _ _ _ _ _ _ _ _ _ _ _]
          dyn-events: _ -> [_ _ _ _ _ _ _ _ _ _ _ _ _]
          timeout: _ -> [_ _ _ _ _ _ _ _ _ _ _ _ _]
          tunnel: [_ _ _ _ _ _ _ _ _ _ _ _ w1223] -> w379
          tunnel: w378 -> [w385 _ w411 _ _ _ _ _ _ _ w864 _ w1216]
          tunnel: w377 -> [_ _ _ _ w435 _ _ _ _ _ _ _ _]
          tunnel: w376 -> [_ _ _ _ w422 w681 w757 w784 w810 w838 _ _ _]
          tunnel: w375 -> [_ _ _ w415 w438 _ _ _ _ _ _ _ _]
          tunnel: w374 -> [_ _ _ _ _ _ _ _ _ _ w853 _ _]
          tunnel: "New Number of Points per Scan" -> [_ _ _ w414 w432 w682 w770 w797 w822 w833 w865 _ _]
          tunnel: "New Scan Frequency (Hz)" -> [_ _ _ _ w433 _ _ _ _ _ w862 _ _]
          tunnel: "New Spacing (um)" -> [_ _ _ _ w431 w680 _ _ w816 w834 w867 _ _]
          tunnel: "New Scan Form" -> [_ _ _ _ w434 _ w771 w798 w821 w832 w866 _ _]
          tunnel: w365 -> [_ _ _ _ _ _ _ _ _ _ _ w1104 _]
          tunnel: w369 -> [_ _ _ _ _ _ _ _ _ _ w863 w1103 _]
          tunnel: w368 -> [_ _ _ _ _ _ _ _ _ _ _ w1102 _]
          tunnel: "New EOD Deflection Scale (um/V)" -> [_ _ _ _ w424 w677 w759 w787 _ w830 w861 _ _]
          tunnel: w366 -> [_ _ _ _ _ _ _ _ _ _ w860 _ _]
          tunnel: [w381 w395 w410 w413 w427 w675 w762 w789 w818 w827 w850 w1101 w1214] -> w364
          tunnel: w363 -> [w381 w395 w410 w413 w427 w675 w762 w789 w818 w827 w849 w1101 w1214]
          tunnel: [w380 w396 w409 w412 w426 w674 w761 w788 w817 w828 w846 w1100 w1213] -> w362
          tunnel: w361 -> [w380 w396 w409 w412 w426 w674 w761 w788 w817 w828 w845 w1100 w1213]
          tunnel: w360 -> [_ _ _ _ _ _ _ _ _ _ _ w1098 _]
          tunnel: w359 -> [_ _ _ _ _ _ _ _ _ _ _ w1099 _]
          tunnel: w358 -> [_ _ _ _ _ _ _ _ _ _ _ w1097 _]
          tunnel: w357 -> [_ _ _ _ _ _ _ _ _ _ w844 _ _]
          tunnel: "New Modulation Radius (um)" -> [_ _ _ _ w423 _ w760 w786 w815 _ w843 _ _]
          tunnel: w355 -> [_ _ _ _ _ _ _ _ _ _ _ w1096 _]
          tunnel: w354 -> [_ _ _ _ _ _ _ _ _ _ _ _ _]
          tunnel: w353 -> [_ _ _ _ _ _ _ _ _ _ _ _ _]
          event "Trap": Value Change {
            # "If Ready (i.e. FPGA has been updated at least once), send a command to start or stop\nIf not Ready, then should not start yet, and no need to stop (since FPGA initializes to off)"
            n160 = event-data() -> ("NewVal"=w384:bool)  [unwired: 1 in]
            n161 = local read "Ready"() -> (w382:bool)
            n162 = And(x=w382, y=w384) -> (x .and. y?=w383:bool)
            n163 = local write "Trap"(w383) -> ()
            n164 = case shown="True" w382 {
              tunnel: w384 -> [_ w388]
              tunnel: w385 -> [_ w387]
              frame False {
              }
              frame True {
                n165 = Join Numbers(hi=u8 1, lo=u8 0) -> ((hi.lo)=w389:u16)
                n166 = Boolean To (0,1)(Boolean=w388) -> (0, 1=w394:i16)
                n167 = Join Numbers(hi=w389, lo=w394) -> ((hi.lo)=w392:u32)
                n168 = Build Array(w392) -> (w393:u32[])
                n169 = xnode "Invoke Method"("FPGA VI Reference In"=w387, "Data"=w393, "Timeout (ms)"=-1) -> ()  [unwired: 1 in, 3 out]
              }
            }
          }
          event "Clear Warnings": Value Change {
            n170 = event-data() -> ()  [unwired: 1 in, 1 out]
            n171 = local write "Unrecognized Command"(FALSE ("Unrecognized Command")) -> ()
            n172 = local write "Photon DMA Overflow"(FALSE ("Photon DMA Overflow")) -> ()
            n173 = local write "On-Chip FIFO Overflow"(FALSE ("On-Chip FIFO Overflow")) -> ()
            n174 = local write "Feedback DMA Overflow"(FALSE ("Feedback DMA Overflow")) -> ()
          }
          event "Include Mobility Update": Value Change {
            n175 = event-data() -> ("NewVal"=w401:bool)  [unwired: 1 in]
            n176 = Join Numbers(hi=u8 4, lo=u8 0) -> ((hi.lo)=w403:u16)
            n177 = Boolean To (0,1)(Boolean=w401) -> (0, 1=w408:i16)
            n178 = Join Numbers(hi=w403, lo=w408) -> ((hi.lo)=w406:u32)
            n179 = Build Array(w406) -> (w407:u32[])
            n180 = xnode "Invoke Method"("FPGA VI Reference In"=w411, "Data"=w407, "Timeout (ms)"=-1) -> ()  [unwired: 1 in, 3 out]
          }
          event "New Scan Frequency (Hz)": Value Change {
            # "Only allow the scan frequency to be changed if it does not max out.\nIf it does max out, then just set the frequency to the maximum allowed."
            n181 = event-data() -> ("NewVal"=w418:dbl)  [unwired: 1 in]
            n182 = Multiply(x=w418, y=w414) -> (x*y=w420:dbl)
            n183 = Less Or Equal?(x=w420, y=w415) -> (x <= y?=w419:bool)
            n184 = Divide(x=w415, y=w414) -> (x/y=w416:dbl)
            n185 = Select(t=w418, s=w419, f=w416) -> (s? t:f=w417:dbl)
            n186 = local write "New Scan Frequency (Hz)"(w417) -> ()
          }
          event "New Number of Points per Scan": Value Change {
            # "Allow the number of points per scan to be changed, as long as\nit does not max out the scan frequency or the maximum voltage"
            n187 = event-data() -> ("NewVal"=w436:u8)  [unwired: 1 in]
            n188 = Divide(x=w423, y=w424) -> (x/y=w425:dbl)
            n189 = Divide(x=w431, y=w424) -> (x/y=w430:dbl)
            n190 = Increment(x=w432) -> (x+1=w440:u8)
            n191 = Equal?(x=w436, y=w440) -> (x = y?=w437:bool)
            n192 = Subtract(x=w422, y=w425) -> (x-y=w421:dbl)
            n193 = case shown="False" w437 {
              tunnel: w434 -> [w449 w569]
              tunnel: [w444 w564] -> w439
              tunnel: w436 -> [w447 w567]
              tunnel: w435 -> [w446 w566]
              tunnel: w430 -> [w448 w568]
              tunnel: w421 -> [w445 w565]
              tunnel: [w443 w563] -> w429
              tunnel: w433 -> [w442 w562]
              tunnel: w438 -> [w441 w561]
              frame False {
                # "Go to largest allowable number of points less than or equal to the requested number of points,\nwithout saturating the Voltage nor the number of points nor the frequency"
                n194 = case shown="\"Square\"" w449 {
                  selector: w449 -> [w454 w484 w521]
                  tunnel: w448 -> [w459 w486 w526]
                  tunnel: w447 -> [w458 w494 w525]
                  tunnel: w446 -> [w457 w493 w524]
                  tunnel: w445 -> [w456 w492 w523]
                  tunnel: [w455 w491 w522] -> w444
                  tunnel: [w451 w488 w518] -> w443
                  tunnel: w442 -> [w453 w490 w520]
                  tunnel: w441 -> [w452 w489 w519]
                  tunnel: [w450 w482 w517] -> _
                  frame "Circular", Default {
                    n195 = while {
                      shift-right: [w463] -> _
                      shift-left: u8 1 -> [w466]
                      tunnel: w459 -> [w481]
                      tunnel: w458 -> [w480]
                      tunnel: w457 -> [w479]
                      tunnel: w456 -> [w478]
                      tunnel: [w466] -> w455
                      tunnel: w454 -> [w473]
                      tunnel: w453 -> [w472]
                      tunnel: w452 -> [w470]
                      shift-right: [w465] -> _
                      shift-left: _ -> [w464]
                      tunnel: [w464] -> w451
                      shift-right: [w462] -> _
                      shift-left: _ -> [w461]
                      tunnel: [w461] -> w450
                      stop <- w474 stop-if-true
                      n196 = Increment(x=w466) -> (x+1=w463:u8)
                      n197 = call "CalculateRadius.vi"("Scan Type"=w473, "Points per Scan"=w463, "Spacing (V)"=w481) -> ("Maximum Voltage (V)"=w462:dbl, "Radius (V)"=w465:dbl)
                      n198 = Greater?(x=w463, y=w479) -> (0:w476:bool)
                      n199 = Multiply(x=w463, y=w472) -> (x*y=w471:dbl)
                      n200 = Greater?(x=w463, y=w480) -> (0:w477:bool)
                      n201 = Greater Or Equal?(x=w462, y=w478) -> (x >= y?=w468:bool)
                      n202 = Greater?(x=w471, y=w470) -> (0:w469:bool)
                      n203 = Or(x=w477, y=w476) -> (x .or. y?=w475:bool)
                      n204 = Or(x=w468, y=w469) -> (x .or. y?=w467:bool)
                      n205 = Or(x=w475, y=w467) -> (x .or. y?=w474:bool)
                    }
                  }
                  frame "Square" {
                    w485 = u8 4
                    n206 = call "CalculateRadius.vi"("Scan Type"=w484, "Points per Scan"=w485, "Spacing (V)"=w486) -> ("Maximum Voltage (V)"=w483:dbl, "Radius (V)"=w487:dbl)
                    n207 = while {
                      shift-right: [w497] -> _
                      shift-left: w485 -> [w507]
                      tunnel: w486 -> [w516]
                      tunnel: w494 -> [w515]
                      tunnel: w493 -> [w514]
                      tunnel: w492 -> [w513]
                      tunnel: [w507] -> w491
                      tunnel: w484 -> [w508]
                      tunnel: w490 -> [w505]
                      tunnel: w489 -> [w503]
                      shift-right: [w499] -> _
                      shift-left: w487 -> [w498]
                      tunnel: [w498] -> w488
                      shift-right: [w496] -> _
                      shift-left: w483 -> [w495]
                      tunnel: [w495] -> w482
                      stop <- w509 stop-if-true
                      n208 = Add(x=w507, y=u8 4) -> (x+y=w497:u8)
                      n209 = call "CalculateRadius.vi"("Scan Type"=w508, "Points per Scan"=w497, "Spacing (V)"=w516) -> ("Maximum Voltage (V)"=w496:dbl, "Radius (V)"=w499:dbl)
                      n210 = Greater?(x=w497, y=w514) -> (0:w511:bool)
                      n211 = Multiply(x=w497, y=w505) -> (x*y=w504:dbl)
                      n212 = Greater?(x=w497, y=w515) -> (0:w512:bool)
                      n213 = Greater Or Equal?(x=w496, y=w513) -> (x >= y?=w501:bool)
                      n214 = Greater?(x=w504, y=w503) -> (0:w502:bool)
                      n215 = Or(x=w512, y=w511) -> (x .or. y?=w510:bool)
                      n216 = Or(x=w501, y=w502) -> (x .or. y?=w500:bool)
                      n217 = Or(x=w510, y=w500) -> (x .or. y?=w509:bool)
                    }
                  }
                  frame "Hexagonal" {
                    n218 = while {
                      shift-right: [w530] -> _
                      shift-left: u8 1 -> [w551]
                      tunnel: w526 -> [w560]
                      tunnel: w525 -> [w559]
                      tunnel: w524 -> [w558]
                      tunnel: w523 -> [w557]
                      tunnel: [w551] -> w522
                      tunnel: w521 -> [w552]
                      tunnel: w520 -> [w550]
                      tunnel: w519 -> [w548]
                      shift-right: [w532] -> _
                      shift-left: _ -> [w531]
                      tunnel: [w531] -> w518
                      shift-right: [w529] -> _
                      shift-left: _ -> [w528]
                      tunnel: [w528] -> w517
                      i -> [w544]
                      stop <- w553 stop-if-true
                      n219 = To Unsigned Byte Integer(number=w544) -> (unsigned 8bit integer=w534:u8)
                      n220 = Multiply(x=w534, y=w534) -> (x*y=w533:u8)
                      n221 = Multiply(x=w534, y=u8 3) -> (x*y=w535:u8)
                      n222 = Add(x=w533, y=w535) -> (x+y=w536:u8)
                      n223 = Add(x=w536, y=u8 2) -> (x+y=w539:u8)
                      n224 = Quotient & Remainder(x=w533, y=u8 4) -> (floor(x/y)=w542:u8)  [unwired: 1 out]
                      n225 = Quotient & Remainder(x=w539, y=u8 2) -> (floor(x/y)=w543:u8)  [unwired: 1 out]
                      n226 = Add(x=w542, y=w543) -> (x+y=w530:u8)
                      n227 = call "CalculateRadius.vi"("Scan Type"=w552, "Points per Scan"=w530, "Spacing (V)"=w560) -> ("Maximum Voltage (V)"=w529:dbl, "Radius (V)"=w532:dbl)
                      n228 = Greater?(x=w530, y=w558) -> (0:w555:bool)
                      n229 = Multiply(x=w530, y=w550) -> (x*y=w549:dbl)
                      n230 = Greater?(x=w530, y=w559) -> (0:w556:bool)
                      n231 = Greater Or Equal?(x=w529, y=w557) -> (x >= y?=w546:bool)
                      n232 = Greater?(x=w549, y=w548) -> (0:w547:bool)
                      n233 = Or(x=w556, y=w555) -> (x .or. y?=w554:bool)
                      n234 = Or(x=w546, y=w547) -> (x .or. y?=w545:bool)
                      n235 = Or(x=w554, y=w545) -> (x .or. y?=w553:bool)
                    }
                  }
                }
              }
              frame True {
                # "Increment to the next allowed number of points, if possible"
                n236 = case shown="\"Circular\", Default" w569 {
                  selector: w569 -> [w572 w600 w634]
                  tunnel: w568 -> [w578 w602 w633]
                  tunnel: w567 -> [w577 w610 w640]
                  tunnel: w566 -> [w576 w609 w639]
                  tunnel: w565 -> [w575 w608 w638]
                  tunnel: [w571 w605 w635] -> w564
                  tunnel: [w570 w604 w632] -> w563
                  tunnel: w562 -> [w574 w607 w637]
                  tunnel: w561 -> [w573 w606 w636]
                  frame "Circular", Default {
                    n237 = while {
                      shift-right: [w581] -> _
                      shift-left: u8 1 -> [w584]
                      tunnel: w578 -> [w599]
                      tunnel: w577 -> [w598]
                      tunnel: w576 -> [w597]
                      tunnel: w575 -> [w596]
                      tunnel: [w584] -> w571
                      tunnel: w572 -> [w591]
                      tunnel: w574 -> [w590]
                      tunnel: w573 -> [w588]
                      shift-right: [w583] -> _
                      shift-left: _ -> [w582]
                      tunnel: [w582] -> w570
                      stop <- w592 stop-if-true
                      n238 = Increment(x=w584) -> (x+1=w581:u8)
                      n239 = call "CalculateRadius.vi"("Scan Type"=w591, "Points per Scan"=w581, "Spacing (V)"=w599) -> ("Maximum Voltage (V)"=w580:dbl, "Radius (V)"=w583:dbl)
                      n240 = Greater?(x=w581, y=w597) -> (0:w594:bool)
                      n241 = Multiply(x=w581, y=w590) -> (x*y=w589:dbl)
                      n242 = Greater Or Equal?(x=w584, y=w598) -> (x >= y?=w595:bool)
                      n243 = Greater Or Equal?(x=w580, y=w596) -> (x >= y?=w586:bool)
                      n244 = Greater?(x=w589, y=w588) -> (0:w587:bool)
                      n245 = Or(x=w595, y=w594) -> (x .or. y?=w593:bool)
                      n246 = Or(x=w586, y=w587) -> (x .or. y?=w585:bool)
                      n247 = Or(x=w593, y=w585) -> (x .or. y?=w592:bool)
                    }
                  }
                  frame "Square" {
                    w601 = u8 4
                    n248 = call "CalculateRadius.vi"("Scan Type"=w600, "Points per Scan"=w601, "Spacing (V)"=w602) -> ("Radius (V)"=w603:dbl)  [unwired: 1 out]
                    n249 = while {
                      shift-right: [w612] -> _
                      shift-left: w601 -> [w615]
                      tunnel: w602 -> [w631]
                      tunnel: w610 -> [w630]
                      tunnel: w609 -> [w629]
                      tunnel: w608 -> [w628]
                      tunnel: [w615] -> w605
                      tunnel: w600 -> [w623]
                      tunnel: w607 -> [w621]
                      tunnel: w606 -> [w619]
                      shift-right: [w614] -> _
                      shift-left: w603 -> [w613]
                      tunnel: [w613] -> w604
                      stop <- w624 stop-if-true
                      n250 = Add(x=w615, y=u8 4) -> (x+y=w612:u8)
                      n251 = call "CalculateRadius.vi"("Scan Type"=w623, "Points per Scan"=w612, "Spacing (V)"=w631) -> ("Maximum Voltage (V)"=w611:dbl, "Radius (V)"=w614:dbl)
                      n252 = Greater?(x=w612, y=w629) -> (0:w626:bool)
                      n253 = Multiply(x=w612, y=w621) -> (x*y=w620:dbl)
                      n254 = Greater Or Equal?(x=w615, y=w630) -> (x >= y?=w627:bool)
                      n255 = Greater Or Equal?(x=w611, y=w628) -> (x >= y?=w617:bool)
                      n256 = Greater?(x=w620, y=w619) -> (0:w618:bool)
                      n257 = Or(x=w627, y=w626) -> (x .or. y?=w625:bool)
                      n258 = Or(x=w617, y=w618) -> (x .or. y?=w616:bool)
                      n259 = Or(x=w625, y=w616) -> (x .or. y?=w624:bool)
                    }
                  }
                  frame "Hexagonal" {
                    n260 = while {
                      shift-right: [w643] -> _
                      shift-left: u8 1 -> [w646]
                      tunnel: w633 -> [w673]
                      tunnel: w640 -> [w672]
                      tunnel: w639 -> [w671]
                      tunnel: w638 -> [w670]
                      tunnel: [w646] -> w635
                      tunnel: w634 -> [w665]
                      tunnel: w637 -> [w664]
                      tunnel: w636 -> [w662]
                      shift-right: [w645] -> _
                      shift-left: _ -> [w644]
                      tunnel: [w644] -> w632
                      i -> [w658]
                      stop <- w666 stop-if-true
                      n261 = To Unsigned Byte Integer(number=w658) -> (unsigned 8bit integer=w647:u8)
                      n262 = Multiply(x=w647, y=w647) -> (x*y=w648:u8)
                      n263 = Multiply(x=w647, y=u8 3) -> (x*y=w649:u8)
                      n264 = Add(x=w648, y=w649) -> (x+y=w650:u8)
                      n265 = Add(x=w650, y=u8 2) -> (x+y=w653:u8)
                      n266 = Quotient & Remainder(x=w648, y=u8 4) -> (floor(x/y)=w656:u8)  [unwired: 1 out]
                      n267 = Quotient & Remainder(x=w653, y=u8 2) -> (floor(x/y)=w657:u8)  [unwired: 1 out]
                      n268 = Add(x=w656, y=w657) -> (x+y=w643:u8)
                      n269 = call "CalculateRadius.vi"("Scan Type"=w665, "Points per Scan"=w643, "Spacing (V)"=w673) -> ("Maximum Voltage (V)"=w642:dbl, "Radius (V)"=w645:dbl)
                      n270 = Greater?(x=w643, y=w671) -> (0:w668:bool)
                      n271 = Multiply(x=w643, y=w664) -> (x*y=w663:dbl)
                      n272 = Greater Or Equal?(x=w646, y=w672) -> (x >= y?=w669:bool)
                      n273 = Greater Or Equal?(x=w642, y=w670) -> (x >= y?=w660:bool)
                      n274 = Greater?(x=w663, y=w662) -> (0:w661:bool)
                      n275 = Or(x=w669, y=w668) -> (x .or. y?=w667:bool)
                      n276 = Or(x=w660, y=w661) -> (x .or. y?=w659:bool)
                      n277 = Or(x=w667, y=w659) -> (x .or. y?=w666:bool)
                    }
                  }
                }
              }
            }
            n278 = Multiply(x=w429, y=w424) -> (x*y=w428:dbl)
            n279 = local write "New Number of Points per Scan"(w439) -> ()
            n280 = local write "New Radius (um)"(w428) -> ()
          }
          event "New Scan Form": Value Change {
            # "Should always end up with fewer points, so no concern about frequency or number of points saturating"
            n281 = event-data() -> ("NewVal"=w683:enum8{"Circular", "Square", "Hexagonal"})  [unwired: 1 in]
            n282 = Divide(x=w680, y=w677) -> (x/y=w679:dbl)
            n283 = case shown="\"Hexagonal\"" w683 {
              selector: w683 -> [w686 w704 w727]
              tunnel: w679 -> [w690 w705 w731]
              tunnel: w682 -> [w689 w711 w730]
              tunnel: w681 -> [w688 w710 w729]
              tunnel: [w687 w709 w728] -> w684
              tunnel: [w685 w708 w725] -> w678
              frame "Circular", Default {
                n284 = while {
                  shift-right: [w697] -> _
                  shift-left: u8 1 -> [w698]
                  tunnel: w690 -> [w703]
                  tunnel: w689 -> [w702]
                  tunnel: w688 -> [w701]
                  tunnel: [w698] -> w687
                  tunnel: w686 -> [w696]
                  shift-right: [w694] -> _
                  shift-left: _ -> [w693]
                  tunnel: [w693] -> w685
                  stop <- w699 stop-if-true
                  n285 = Increment(x=w698) -> (x+1=w697:u8)
                  n286 = call "CalculateRadius.vi"("Scan Type"=w696, "Points per Scan"=w697, "Spacing (V)"=w703) -> ("Maximum Voltage (V)"=w692:dbl, "Radius (V)"=w694:dbl)
                  n287 = Greater?(x=w697, y=w702) -> (0:w695:bool)
                  n288 = Greater Or Equal?(x=w692, y=w701) -> (x >= y?=w700:bool)
                  n289 = Or(x=w695, y=w700) -> (x .or. y?=w699:bool)
                }
              }
              frame "Square" {
                w706 = u8 4
                n290 = call "CalculateRadius.vi"("Scan Type"=w704, "Points per Scan"=w706, "Spacing (V)"=w705) -> ("Radius (V)"=w707:dbl)  [unwired: 1 out]
                n291 = while {
                  shift-right: [w717] -> _
                  shift-left: w706 -> [w718]
                  tunnel: w705 -> [w724]
                  tunnel: w711 -> [w723]
                  tunnel: w710 -> [w722]
                  tunnel: [w718] -> w709
                  tunnel: w704 -> [w719]
                  shift-right: [w714] -> _
                  shift-left: w707 -> [w713]
                  tunnel: [w713] -> w708
                  stop <- w720 stop-if-true
                  n292 = Add(x=w718, y=u8 4) -> (x+y=w717:u8)
                  n293 = call "CalculateRadius.vi"("Scan Type"=w719, "Points per Scan"=w717, "Spacing (V)"=w724) -> ("Maximum Voltage (V)"=w712:dbl, "Radius (V)"=w714:dbl)
                  n294 = Greater?(x=w717, y=w723) -> (0:w715:bool)
                  n295 = Greater Or Equal?(x=w712, y=w722) -> (x >= y?=w721:bool)
                  n296 = Or(x=w715, y=w721) -> (x .or. y?=w720:bool)
                }
              }
              frame "Hexagonal" {
                n297 = while {
                  shift-right: [w734] -> _
                  shift-left: u8 1 -> [w749]
                  tunnel: w731 -> [w755]
                  tunnel: w730 -> [w754]
                  tunnel: w729 -> [w753]
                  tunnel: [w749] -> w728
                  tunnel: w727 -> [w750]
                  shift-right: [w747] -> _
                  shift-left: _ -> [w745]
                  tunnel: [w745] -> w725
                  i -> [w748]
                  stop <- w751 stop-if-true
                  n298 = To Unsigned Byte Integer(number=w748) -> (unsigned 8bit integer=w733:u8)
                  n299 = Multiply(x=w733, y=w733) -> (x*y=w735:u8)
                  n300 = Multiply(x=w733, y=u8 3) -> (x*y=w736:u8)
                  n301 = Add(x=w735, y=w736) -> (x+y=w737:u8)
                  n302 = Add(x=w737, y=u8 2) -> (x+y=w740:u8)
                  n303 = Quotient & Remainder(x=w735, y=u8 4) -> (floor(x/y)=w743:u8)  [unwired: 1 out]
                  n304 = Quotient & Remainder(x=w740, y=u8 2) -> (floor(x/y)=w744:u8)  [unwired: 1 out]
                  n305 = Add(x=w743, y=w744) -> (x+y=w734:u8)
                  n306 = call "CalculateRadius.vi"("Scan Type"=w750, "Points per Scan"=w734, "Spacing (V)"=w755) -> ("Maximum Voltage (V)"=w732:dbl, "Radius (V)"=w747:dbl)
                  n307 = Greater?(x=w734, y=w754) -> (0:w746:bool)
                  n308 = Greater Or Equal?(x=w732, y=w753) -> (x >= y?=w752:bool)
                  n309 = Or(x=w746, y=w752) -> (x .or. y?=w751:bool)
                }
              }
            }
            n310 = Multiply(x=w678, y=w677) -> (x*y=w676:dbl)
            n311 = local write "New Number of Points per Scan"(w684) -> ()
            n312 = local write "New Radius (um)"(w676) -> ()
          }
          event "New Spacing (um)": Value Change {
            # "Allow the spacing between points to change as long\nas it does not saturate the maximum voltage applied"
            n313 = event-data() -> ("NewVal"=w768:dbl)  [unwired: 1 in]
            n314 = Divide(x=w760, y=w759) -> (x/y=w758:dbl)
            n315 = Divide(x=w768, y=w759) -> (x/y=w767:dbl)
            n316 = call "CalculateRadius.vi"("Scan Type"=w771, "Points per Scan"=w770, "Spacing (V)"=w767) -> ("Maximum Voltage (V)"=w769:dbl, "Radius (V)"=w772:dbl)
            n317 = Subtract(x=w757, y=w758) -> (x-y=w756:dbl)
            n318 = Less Or Equal?(x=w756, y=w769) -> (x <= y?=w773:bool)
            n319 = case shown="True" w773 {
              tunnel: w756 -> [_ w782]
              tunnel: w769 -> [_ w781]
              tunnel: w772 -> [w775 w780]
              tunnel: w767 -> [w774 w778]
              tunnel: [w775 w777] -> w765
              tunnel: [w774 w776] -> w766
              frame False {
                # "Not oversaturated"
              }
              frame True {
                # "Oversaturated"
                n320 = Divide(x=w782, y=w781) -> (x/y=w779:dbl)
                n321 = Multiply(x=w779, y=w778) -> (x*y=w776:dbl)
                n322 = Multiply(x=w779, y=w780) -> (x*y=w777:dbl)
              }
            }
            n323 = Multiply(x=w766, y=w759) -> (x*y=w763:dbl)
            n324 = Multiply(x=w765, y=w759) -> (x*y=w764:dbl)
            n325 = local write "New Spacing (um)"(w763) -> ()
            n326 = local write "New Radius (um)"(w764) -> ()
          }
          event "New Radius (um)": Value Change {
            # "Allow the radius of the pattern to change as long\nas it does not saturate the maximum voltage applied"
            n327 = event-data() -> ()  [unwired: 1 in, 1 out]
            n328 = Divide(x=w786, y=w787) -> (x/y=w785:dbl)
            n329 = Divide(x="New Radius (um)", y=w787) -> (x/y=w794:dbl)
            n330 = Subtract(x=w784, y=w785) -> (x-y=w783:dbl)
            n331 = call "CalculateSpacing.vi"("Scan Type"=w798, "Points per Scan"=w797, "Radius (V)"=w794) -> ("Maximum Voltage (V)"=w796:dbl, "Spacing (V)"=w799:dbl)
            n332 = Less Or Equal?(x=w783, y=w796) -> (x <= y?=w800:bool)
            n333 = case shown="True" w800 {
              tunnel: w783 -> [_ w809]
              tunnel: w796 -> [_ w808]
              tunnel: w799 -> [w802 w807]
              tunnel: w794 -> [w801 w805]
              tunnel: [w802 w804] -> w792
              tunnel: [w801 w803] -> w793
              frame False {
                # "Not oversaturated"
              }
              frame True {
                # "Oversaturated"
                n334 = Divide(x=w809, y=w808) -> (x/y=w806:dbl)
                n335 = Multiply(x=w806, y=w805) -> (x*y=w803:dbl)
                n336 = Multiply(x=w806, y=w807) -> (x*y=w804:dbl)
              }
            }
            n337 = Multiply(x=w793, y=w787) -> (x*y=w791:dbl)
            n338 = Multiply(x=w792, y=w787) -> (x*y=w790:dbl)
            n339 = local write "New Spacing (um)"(w790) -> ()
            n340 = local write "New Radius (um)"(w791) -> ()
          }
          event "New EOD Deflection Scale (um/V)": Value Change {
            n341 = event-data() -> ("NewVal"=w813:dbl)  [unwired: 1 in]
            n342 = call "CalculateRadius.vi"("Scan Type"=w821, "Points per Scan"=w822, "Spacing (V)"=w816) -> ("Maximum Voltage (V)"=w814:dbl)  [unwired: 1 out]
            n343 = Add(x=w815, y=w814) -> (x+y=w812:dbl)
            n344 = Multiply(x=w810, y=w813) -> (x*y=w811:dbl)
            n345 = Less Or Equal?(x=w811, y=w812) -> (x <= y?=w820:bool)
            n346 = case shown="True" w820 {
              tunnel: w813 -> [w823 _]
              tunnel: [w823 w826] -> w819
              tunnel: w812 -> [_ w825]
              tunnel: w810 -> [_ w824]
              frame False {
              }
              frame True {
                # "Oversaturated"
                n347 = Divide(x=w824, y=w825) -> (x/y=w826:dbl)
              }
            }
            n348 = local write "New EOD Deflection Scale (um/V)"(w819) -> ()
          }
          event "New Modulation Radius (um)": Value Change {
            n349 = event-data() -> ("NewVal"=w837:dbl)  [unwired: 1 in]
            n350 = Divide(x=w837, y=w830) -> (x/y=w836:dbl)
            n351 = Divide(x=w834, y=w830) -> (x/y=w835:dbl)
            n352 = call "CalculateRadius.vi"("Scan Type"=w832, "Points per Scan"=w833, "Spacing (V)"=w835) -> ("Maximum Voltage (V)"=w839:dbl)  [unwired: 1 out]
            n353 = Add(x=w839, y=w836) -> (x+y=w841:dbl)
            n354 = Less?(x=w841, y=w838) -> (x < y?=w842:bool)
            n355 = Subtract(x=w838, y=w839) -> (x-y=w840:dbl)
            n356 = Select(t=w836, s=w842, f=w840) -> (s? t:f=w831:dbl)
            n357 = Multiply(x=w831, y=w830) -> (x*y=w829:dbl)
            n358 = local write "New Modulation Radius (um)"(w829) -> ()
          }
          event "Update FPGA": Value Change {
            n359 = event-data() -> ()  [unwired: 1 in, 1 out]
            n360 = flat-sequence {
              tunnel: [w890] -> w859
              tunnel: w865 -> [w890]
              tunnel: w864 -> [w897]
              tunnel: [w896] -> w858
              tunnel: w863 -> [w895]
              tunnel: w862 -> [w891]
              tunnel: [w894] -> w857
              tunnel: w853 -> [w880]
              tunnel: [w880] -> w852
              tunnel: [w879] -> w851
              tunnel: [w879] -> w850
              tunnel: w849 -> [w889]
              tunnel: [w876] -> w848
              tunnel: [w875] -> w847
              tunnel: [w874] -> w846
              tunnel: w845 -> [w873]
              tunnel: w844 -> [w868]
              tunnel: [w945] -> w856
              tunnel: w867 -> [w1006]
              tunnel: w866 -> [w1033]
              tunnel: w859 -> [w972]
              tunnel: w858 -> [w1038]
              tunnel: [w1038] -> w855
              tunnel: w861 -> [w922]
              tunnel: w860 -> [w997]
              tunnel: w857 -> [w1002]
              tunnel: [w1002] -> w854
              tunnel: w852 -> [w990]
              tunnel: w851 -> [w967]
              tunnel: w848 -> [w989]
              tunnel: w847 -> [w988]
              tunnel: w843 -> [w926]
              tunnel: w856 -> [w1084]
              tunnel: w855 -> [w1085]
              tunnel: w854 -> [w1082]
              frame #0 {
                # "Bin Length (ticks)"
                n361 = Multiply(x=w891, y=w890) -> (x*y=w893:dbl)
                n362 = Divide(x=w880, y=w893) -> (x/y=w892:dbl)
                n363 = To Unsigned Word Integer(number=w892) -> (unsigned 16bit integer=w879:u16)
                n364 = Square(x="New Beam Waist Estimate (um)") -> (x^2=w888:dbl)
                n365 = Multiply(x=u16 2, y=w879) -> (x*y=w881:u16)
                n366 = Multiply(x=w880, y=w888) -> (x*y=w884:dbl)
                n367 = Multiply(x="New Diffusion Constant Estimate (um^2/s)", y=w881) -> (x*y=w887:dbl)
                n368 = Divide(x=w884, y=w887) -> (x/y=w872:dbl)
                n369 = Scale By Power Of 2(n=w868, x=w872) -> (x*2^n=w871:dbl)
                n370 = To Unsigned Long Integer(number=w871) -> (unsigned 32bit integer=w885:u32)
                n371 = Split Number(x=w885) -> (hi(x)=w886:u16, lo(x)=w875:u16)
                n372 = local read "Trap"() -> (w894:bool)
                n373 = Split Number(x=w886) -> (lo(x)=w876:u8)  [unwired: 1 out]
                n374 = Join Numbers(hi=w876, lo=w875) -> ((hi.lo)=w874:u32)
                n375 = Multiply(x=w874, y=w881) -> (x*y=w882:u32)
                n376 = case shown="True" w894 {
                  tunnel: w897 -> [w898 w911]
                  tunnel: [w898 w910] -> w896
                  tunnel: w890 -> [_ w905]
                  tunnel: w895 -> [_ w909]
                  tunnel: w879 -> [_ w908]
                  tunnel: w874 -> [_ w904]
                  tunnel: w873 -> [_ w903]
                  tunnel: w889 -> [_ w900]
                  frame False {
                  }
                  frame True {
                    n377 = Not Equal?(x=w904, y=w903) -> (x != y?=w899:bool)
                    n378 = Not Equal?(x=w909, y=w905) -> (x != y?=w906:bool)
                    n379 = Not Equal?(x=w900, y=w908) -> (x != y?=w907:bool)
                    n380 = Or(x=w906, y=w907) -> (x .or. y?=w902:bool)
                    n381 = Or(x=w899, y=w902) -> (x .or. y?=w901:bool)
                    n382 = case shown="True" w901 {
                      tunnel: w911 -> [w912 w920]
                      tunnel: [w912 w913] -> w910
                      frame False {
                      }
                      frame True {
                        # "Critical parameter change - must stop during update"
                        n383 = Join Numbers(hi=u8 1, lo=u8 0) -> ((hi.lo)=w917:u16)
                        n384 = Join Numbers(hi=w917, lo=u16 0) -> ((hi.lo)=w915:u32)
                        n385 = Build Array(w915) -> (w914:u32[])
                        n386 = xnode "Invoke Method"("FPGA VI Reference In"=w920, "Data"=w914) -> ("FPGA VI Reference Out"=w913:refnum<k20>)  [unwired: 2 in, 2 out]
                      }
                    }
                  }
                }
                n387 = Divide(x=w884, y=w882) -> (x/y=w870:dbl)
                n388 = Scale By Power Of 2(n=w868, x=w870) -> (x*2^n=→"Current Diffusion Constant Estimate (um^2/s)":dbl)
                "Current Beam Waist Estimate (um)" <- "New Beam Waist Estimate (um)"
              }
              frame #1 {
                w942 = 3276.8 ("y")
                w970 = 3276.8 ("y")
                w1035 = 3276.8 ("y")
                # "Modulation points"
                # "EOD positions"
                # "Determine the Voltages required for the requested pattern/number of points"
                n389 = To Double Precision Float(number=w967) -> (double precision float=w966:dbl)
                n390 = Multiply(x=w966, y=w972) -> (x*y=w1039:dbl)
                n391 = Multiply(x=w990, y=w922) -> (x*y=w1000:dbl)
                n392 = Divide(x=w990, y=w1039) -> (x/y=w961:dbl)
                "Current Scan Frequency (Hz)" <- w961
                n393 = Initialize Array "Commands to Send"(u32 0 ("element"), 0 ("dimension size")) -> (w1042:u32[])
                n394 = To Unsigned Word Integer(number=w972) -> (unsigned 16bit integer=w998:u16)
                n395 = Join Numbers(hi=u8 8, lo=u8 0) -> ((hi.lo)=w1027:u16)
                n396 = Join Numbers(hi=w1027, lo=w967) -> ((hi.lo)=w1024:u32)
                n397 = Multiply(x="New Number of Modulation Points", y="New Modulation Frequency (Hz)") -> (x*y=w964:dbl)
                n398 = Insert Into Array "Bin Length"(array=w1042, new element=w1024) -> (w1041:u32[])  [unwired: 1 in]
                n399 = Divide(x=w961, y=w964) -> (x/y=w963:dbl)
                n400 = To Unsigned Long Integer(number=w963) -> (unsigned 32bit integer=w954:u32)
                n401 = Join Numbers(hi=u8 9, lo=u8 0) -> ((hi.lo)=w1023:u16)
                n402 = Split Number(x=w954) -> (hi(x)=w958:u16, lo(x)=w929:u16)
                n403 = Join Numbers(hi=w1023, lo=w998) -> ((hi.lo)=w1020:u32)
                n404 = Split Number(x=w958) -> (lo(x)=w930:u8)  [unwired: 1 out]
                n405 = Join Numbers(hi=u8 0, lo=w930) -> ((hi.lo)=w931:u16)
                n406 = Insert Into Array "Bins/cycle"(array=w1041, new element=w1020) -> (w1040:u32[])  [unwired: 1 in]
                n407 = Join Numbers(hi=w931, lo=w929) -> ((hi.lo)=w927:u32)
                n408 = Multiply(x="New Number of Modulation Points", y=w927) -> (x*y=w962:u32)
                n409 = Join Numbers(hi=u8 11, lo=u8 0) -> ((hi.lo)=w1017:u16)
                n410 = Divide(x=w961, y=w962) -> (x/y=→"Current Modulation Frequency (Hz)":dbl)
                n411 = Join Numbers(hi=w1017, lo="New Sub-Bin Delay") -> ((hi.lo)=w1016:u32)
                n412 = Multiply(x="New Mobility Estimate (um/s/V)", y=w966) -> (x*y=w1009:dbl)
                n413 = Divide(x=w1000, y=w1009) -> (x/y=w1008:dbl)
                n414 = Insert Into Array "Sub-Bin Delay"(array=w1040, new element=w1016) -> (w1029:u32[])  [unwired: 1 in]
                n415 = To Word Integer(number=w1008) -> (16bit integer=w980:i16)
                n416 = Join Numbers(hi=u8 5, lo=w989) -> ((hi.lo)=w1014:u16)
                n417 = Join Numbers(hi=w1014, lo=w988) -> ((hi.lo)=w1013:u32)
                n418 = In Range and Coerce(upper limit=i16 32767, x=w980, lower limit=i16 -32767) -> (coerced(x)=w976:i16)  [unwired: 1 out]
                n419 = Insert Into Array "Inverse Diffusion Constant"(array=w1029, new element=w1013) -> (w1028:u32[])  [unwired: 1 in]
                n420 = Multiply(x=w976, y=w966) -> (x*y=w999:dbl)
                n421 = Absolute Value(x=w976) -> (abs(x)=w973:i16)
                n422 = Join Numbers(hi=u8 6, lo=u8 0) -> ((hi.lo)=w1011:u16)
                n423 = Multiply(x=w970, y="New Maximum Feedback (V)") -> (x*y=w969:dbl)
                n424 = Divide(x=w1000, y=w999) -> (x/y=→"Current Mobility Estimate (um/s/V)":dbl)
                n425 = Join Numbers(hi=w1011, lo=w976) -> ((hi.lo)=w1010:u32)
                n426 = To Word Integer(number=w969) -> (16bit integer=w968:i16)
                n427 = Insert Into Array "Inverse Mobility"(array=w1028, new element=w1010) -> (w993:u32[])  [unwired: 1 in]
                n428 = Quotient & Remainder(x=w968, y=w973) -> (floor(x/y)=w977:i16)  [unwired: 1 out]
                n429 = call "CreateScanPattern.vi"("Point Spacing"=w1006, "Number of Points"=w972, "Pattern"=w1033) -> ("Radius"=→"Current Radius (um)":dbl, "Y coordinates"=w1031:dbl[], "X coordinates"=w1030:dbl[])
                n430 = Multiply(x=w977, y=w973) -> (x*y=w975:i16)
                n431 = Join Numbers(hi=u8 7, lo=u8 0) -> ((hi.lo)=w995:u16)
                n432 = Join Numbers(hi=w995, lo=w977) -> ((hi.lo)=w996:u32)
                n433 = Insert Into Array "Saturated Position Step"(array=w993, new element=w996) -> (w983:u32[])  [unwired: 1 in]
                n434 = Bundle("X coordinates"=w1030, "Y coordinates"=w1031) -> (w933:T5)  [unwired: 1 in]
                n435 = Build Array(w1030, w1031) -> (w1005:dbl[][])
                n436 = Divide(x=w1005, y=w922) -> (x/y=w1004:dbl[][])
                n437 = Divide(x=w975, y=w970) -> (x/y=→"Current Maximum Feedback (V)":dbl)
                n438 = Multiply(x=w1004, y=w1035) -> (x*y=w1036:dbl[][])
                n439 = Join Numbers(hi=u8 4, lo=u8 0) -> ((hi.lo)=w984:u16)
                n440 = Boolean To (0,1)(Boolean="Include Mobility Update") -> (0, 1=w987:i16)
                n441 = To Word Integer(number=w1036) -> (16bit integer=w1003:i16[][])
                n442 = Join Numbers(hi=w984, lo=w987) -> ((hi.lo)=w982:u32)
                n443 = Divide(x=w1003, y=w1035) -> (x/y=w1034:dbl[][])
                n444 = local write "Current Voltages"(w1034) -> ()
                n445 = Insert Into Array "Include Mobility Update"(array=w983, new element=w982) -> (w959:u32[])  [unwired: 1 in]
                n446 = call "InterpolateCircle.vi"("Radius"=w926, "Start Angle (degrees)"="New Modulation Angle (degrees)", "Number of Points"="New Number of Modulation Points") -> ("Y coordinates"=w935:dbl[], "X coordinates"=w936:dbl[])
                n447 = Join Numbers(hi=u8 12, lo=w930) -> ((hi.lo)=w956:u16)
                n448 = Join Numbers(hi=w956, lo=w929) -> ((hi.lo)=w955:u32)
                n449 = Bundle("X coordinates"=w936, "Y coordinates"=w935) -> (w934:T5)  [unwired: 1 in]
                n450 = Build Array(w936, w935) -> (w925:dbl[][])
                n451 = Insert Into Array "Cycles per Modulation Point"(array=w959, new element=w955) -> (w949:u32[])  [unwired: 1 in]
                n452 = Divide(x=w925, y=w922) -> (x/y=w924:dbl[][])
                n453 = Build Array(w933, w934) -> (w932:T1)
                n454 = case shown="False" w1002 {
                  tunnel: w932 -> [w1063 _]
                  frame False {
                    n455 = local write "Position Plot"(w1063) -> ()
                  }
                  frame True {
                  }
                }
                n456 = Multiply(x=w924, y=w942) -> (x*y=w944:dbl[][])
                n457 = Join Numbers(hi=u8 13, lo=u8 0) -> ((hi.lo)=w952:u16)
                n458 = Join Numbers(hi=w952, lo="New Number of Modulation Points") -> ((hi.lo)=w951:u32)
                n459 = To Word Integer(number=w944) -> (16bit integer=w943:i16[][])
                n460 = Insert Into Array "Number of Modulation Points"(array=w949, new element=w951) -> (w947:u32[])  [unwired: 1 in]
                n461 = Divide(x=w943, y=w942) -> (x/y=w941:dbl[][])
                "Current Modulation Voltages" <- w941
                n462 = for {
                  N: w972 -> [_]
                  shift-right: [w1068] -> w946
                  shift-left: w947 -> [w1069]
                  tunnel: w1003 -> [w1067]
                  i -> [w1065]
                  n463 = Index Array(array=w1067, index (col)=w1065) -> (element=w1066:i16[])  [unwired: 1 in]
                  n464 = for {
                    N: 2 -> [_]
                    tunnel: w1066 -> [w1070] mode=indexing
                    tunnel: w1065 -> [w1079]
                    shift-right: [w1073] -> w1068
                    shift-left: w1069 -> [w1074]
                    i -> [w1081]
                    n465 = To Unsigned Byte Integer(number=w1079) -> (unsigned 8bit integer=w1078:u8)
                    n466 = To Unsigned Byte Integer(number=w1081) -> (unsigned 8bit integer=w1071:u8)
                    n467 = Add(x=w1071, y=u8 16 ("x")) -> (x+y=w1080:u8)
                    n468 = Join Numbers(hi=w1080, lo=w1078) -> ((hi.lo)=w1077:u16)
                    n469 = To Unsigned Word Integer(number=w1070) -> (unsigned 16bit integer=w1076:u16)
                    n470 = Join Numbers(hi=w1077, lo=w1076) -> ((hi.lo)=w1075:u32)
                    n471 = Insert Into Array(array=w1074, new element=w1075) -> (w1073:u32[])  [unwired: 1 in]
                  }
                }
                n472 = Square(x=w941) -> (x^2=w940:dbl[][])
                n473 = Add Array Elements(numeric array=w940) -> (sum=w939:dbl)
                n474 = Divide(x=w939, y="New Number of Modulation Points") -> (x/y=w937:dbl)
                n475 = Send Notification(notification=w932, notifier=w997) -> ()  [unwired: 1 in, 2 out]
                n476 = Square Root(x=w937) -> (sqrt(x)=w923:dbl)
                n477 = Multiply(x=w923, y=w922) -> (x*y=→"Current Modulation Radius (um)":dbl)
                n478 = for {
                  N: "New Number of Modulation Points" -> [_]
                  shift-right: [w1049] -> w945
                  shift-left: w946 -> [w1050]
                  tunnel: w943 -> [w1048]
                  i -> [w1046]
                  n479 = Index Array(array=w1048, index (col)=w1046) -> (element=w1047:i16[])  [unwired: 1 in]
                  n480 = for {
                    N: 2 -> [_]
                    tunnel: w1047 -> [w1051] mode=indexing
                    tunnel: w1046 -> [w1060]
                    shift-right: [w1054] -> w1049
                    shift-left: w1050 -> [w1055]
                    i -> [w1062]
                    n481 = To Unsigned Byte Integer(number=w1060) -> (unsigned 8bit integer=w1059:u8)
                    n482 = To Unsigned Byte Integer(number=w1062) -> (unsigned 8bit integer=w1052:u8)
                    n483 = Add(x=w1052, y=u8 20 ("x")) -> (x+y=w1061:u8)
                    n484 = Join Numbers(hi=w1061, lo=w1059) -> ((hi.lo)=w1058:u16)
                    n485 = To Unsigned Word Integer(number=w1051) -> (unsigned 16bit integer=w1057:u16)
                    n486 = Join Numbers(hi=w1058, lo=w1057) -> ((hi.lo)=w1056:u32)
                    n487 = Insert Into Array(array=w1055, new element=w1056) -> (w1054:u32[])  [unwired: 1 in]
                  }
                }
                "Current Scan Form" <- w1033
                "Current Spacing (um)" <- w1006
                "Current EOD Deflection Scale (um/V)" <- w922
                "Current Sub-Bin Delay" <- "New Sub-Bin Delay"
                "Current Number of Points per Scan" <- w972
                "Current Number of Modulation Points" <- "New Number of Modulation Points"
                "Current Modulation Angle (degrees)" <- "New Modulation Angle (degrees)"
              }
              frame #2 {
                n488 = case shown="True" w1082 {
                  tunnel: w1084 -> [w1088 w1091]
                  tunnel: [w1088 w1090] -> w1083
                  frame False {
                  }
                  frame True {
                    # "Restart things (if going)"
                    n489 = Join Numbers(hi=u8 1, lo=u8 0) -> ((hi.lo)=w1093:u16)
                    n490 = Join Numbers(hi=w1093, lo=u16 1) -> ((hi.lo)=w1089:u32)
                    n491 = Insert Into Array(array=w1091, new element=w1089) -> (w1090:u32[])  [unwired: 1 in]
                  }
                }
                n492 = xnode "Invoke Method"("FPGA VI Reference In"=w1085, "Data"=w1083, "Timeout (ms)"=-1) -> ()  [unwired: 1 in, 3 out]
                n493 = local write "Ready"(TRUE ("Ready")) -> ()
              }
            }
          }
          event "Record": Value Change {
            n494 = event-data() -> ("NewVal"=w1105:bool)  [unwired: 1 in]
            n495 = case shown="True" w1105 {
              tunnel: w1104 -> [_ w1119]
              tunnel: w1103 -> [_ w1118]
              tunnel: w1102 -> [w1109 w1120]
              tunnel: w1099 -> [_ w1116]
              tunnel: w1098 -> [_ w1115]
              tunnel: w1097 -> [_ w1114]
              tunnel: w1096 -> [_ w1113]
              frame False {
                # "Close any file created previously if it hasn't been used"
                n496 = Wait on Notification(notifier=w1109, timeout in ms (-1)=0) -> (notification=w1106:T2, timed out?=w1107:bool)  [unwired: 2 in, 2 out]
                n497 = case shown="False" w1107 {
                  tunnel: w1106 -> [w1112 _]
                  frame False {
                    n498 = Unbundle(w1112) -> ("Photon File"=w1111:refnum<file>, "Feedback File"=w1110:refnum<file>)
                    n499 = Close File(refnum=w1110) -> ()  [unwired: 1 in, 2 out]
                    n500 = Close File(refnum=w1111) -> ()  [unwired: 1 in, 2 out]
                  }
                  frame True {
                  }
                }
              }
              frame True {
                n501 = local read "Trap"() -> (w1117:bool)
                n502 = case shown="True" w1117 {
                  tunnel: w1120 -> [_ w1131]
                  tunnel: w1119 -> [_ w1130]
                  tunnel: w1118 -> [_ w1129]
                  tunnel: w1116 -> [w1121 _]
                  tunnel: w1115 -> [_ w1125]
                  tunnel: w1114 -> [_ w1124]
                  tunnel: w1113 -> [_ w1123]
                  frame False {
                    # "Not in any data-acquisition mode - cannot record"
                    n503 = local write "Record"(FALSE ("Record")) -> ()
                    n504 = One Button Dialog(message=w1121) -> ()  [unwired: 1 in, 1 out]
                  }
                  frame True {
                    n505 = Build Path(base path="Top-Level Folder", name or relative path="Prefix") -> (appended path=w1126:path)
                    n506 = call <vilib>:"Check if File or Folder Exists.vi"("path"=w1126) -> ("file or folder exists?"=w1128:bool)  [unwired: 8 in, 2 out]
                    n507 = case shown="False" w1128 {
                      tunnel: w1131 -> [w1188 _]
                      tunnel: w1130 -> [w1177 _]
                      tunnel: w1129 -> [w1175 _]
                      tunnel: "Prefix" -> [w1139 _]
                      tunnel: w1126 -> [w1161 _]
                      tunnel: w1125 -> [_ w1212]
                      tunnel: w1124 -> [w1158 _]
                      tunnel: w1123 -> [w1138 _]
                      frame False {
                        # "Modulation Text Header File"
                        # "Modulation Binary Header File (Voltages lookup tables)"
                        # "Binary Header File (Voltages lookup tables)"
                        # "Binary Data Files"
                        # "Text Header File"
                        # "Open files and output header information"
                        n508 = local read "Current Sub-Bin Delay"() -> (w1171:u16)
                        n509 = local read "Current Diffusion Constant Estimate (um^2/s)"() -> (w1174:dbl)
                        n510 = Multiply(x=w1177, y=w1175) -> (x*y=w1201:dbl)
                        n511 = local read "Current Number of Modulation Points"() -> (w1136:u8)
                        n512 = local read "Current EOD Deflection Scale (um/V)"() -> (w1178:dbl)
                        n513 = local read "Current Modulation Frequency (Hz)"() -> (w1137:dbl)
                        n514 = Divide(x=1000000000.0, y=w1201) -> (x/y=w1182:dbl)
                        n515 = local read "Current Mobility Estimate (um/s/V)"() -> (w1173:dbl)
                        n516 = local read "Current Beam Waist Estimate (um)"() -> (w1179:dbl)
                        n517 = local read "Current Modulation Radius (um)"() -> (w1134:dbl)
                        n518 = local read "Current Maximum Feedback (V)"() -> (w1159:dbl)
                        n519 = local read "Current Modulation Angle (degrees)"() -> (w1135:dbl)
                        n520 = Divide(x=w1171, y=0.08 ("x")) -> (x/y=w1180:dbl)
                        n521 = local read "Include Mobility Update"() -> (w1160:bool)
                        n522 = local read "Current Spacing (um)"() -> (w1181:dbl)
                        n523 = local read "Current Scan Form"() -> (w1170:enum8{"Circular", "Square", "Hexagonal"})
                        n524 = Get Date/Time In Seconds() -> (seconds since 1Jan1904=w1203:timestamp)
                        n525 = Format Date/Time String(time format string (%c)="%Y-%m-%d\n%H:%M:%S\n", seconds (now)=w1203) -> (date/time string=w1183:string)  [unwired: 1 in]
                        n526 = Format Into String(format string=w1158, initial string=w1183, w1177, w1182, w1170, w1175, w1181, w1180, w1179, w1178, w1174, w1173, w1159, w1160) -> (resulting string=w1172:string)  [unwired: 1 in, 1 out]
                        n527 = Format Into String(format string=w1138, w1137, w1136, w1134, w1135) -> (resulting string=w1133:string)  [unwired: 2 in, 1 out]
                        n528 = local read "Current Modulation Voltages"() -> (w1148:dbl[][])
                        n529 = local read "Current Voltages"() -> (w1184:dbl[][])
                        n530 = Create Folder(path (use dialog)=w1161) -> (created path=w1140:path)  [unwired: 2 in, 2 out]
                        n531 = Concatenate Strings(w1139, "_modheader.txt" ("string")) -> (w1142:string)
                        n532 = Concatenate Strings(w1139, "_header.dat" ("string")) -> (w1209:string)
                        n533 = Concatenate Strings(w1139, "_header.txt" ("string")) -> (w1197:string)
                        n534 = Concatenate Strings(w1139, "_modheader.dat" ("string")) -> (w1149:string)
                        n535 = Concatenate Strings(w1139, "_photons.dat" ("string")) -> (w1204:string)
                        n536 = Concatenate Strings(w1139, "_feedbacks.dat" ("string")) -> (w1166:string)
                        n537 = Build Path(base path=w1140, name or relative path=w1149) -> (appended path=w1156:path)
                        n538 = Build Path(base path=w1140, name or relative path=w1142) -> (appended path=w1145:path)
                        n539 = Build Path(base path=w1140, name or relative path=w1209) -> (appended path=w1208:path)
                        n540 = Build Path(base path=w1140, name or relative path=w1197) -> (appended path=w1194:path)
                        n541 = Build Path(base path=w1140, name or relative path=w1204) -> (appended path=w1189:path)
                        n542 = Build Path(base path=w1140, name or relative path=w1166) -> (appended path=w1169:path)
                        n543 = Open/Create/Replace File(file path (use dialog)=w1156, operation (0:open)=T4."create", access (0:read/write)=enum16{"read/write", "read-only", "write-only"}."write-only") -> (refnum out=w1153:refnum<file>)  [unwired: 3 in, 2 out]
                        n544 = Open/Create/Replace File(file path (use dialog)=w1145, operation (0:open)=T4."create", access (0:read/write)=enum16{"read/write", "read-only", "write-only"}."write-only") -> (refnum out=w1147:refnum<file>)  [unwired: 3 in, 2 out]
                        n545 = Open/Create/Replace File(file path (use dialog)=w1194, operation (0:open)=T4."create", access (0:read/write)=enum16{"read/write", "read-only", "write-only"}."write-only") -> (refnum out=w1192:refnum<file>)  [unwired: 3 in, 2 out]
                        n546 = Open/Create/Replace File(file path (use dialog)=w1189, operation (0:open)=T4."create", access (0:read/write)=enum16{"read/write", "read-only", "write-only"}."write-only") -> (refnum out=w1164:refnum<file>)  [unwired: 3 in, 2 out]
                        n547 = Open/Create/Replace File(file path (use dialog)=w1169, operation (0:open)=T4."create", access (0:read/write)=enum16{"read/write", "read-only", "write-only"}."write-only") -> (refnum out=w1163:refnum<file>)  [unwired: 3 in, 2 out]
                        n548 = Open/Create/Replace File(file path (use dialog)=w1208, operation (0:open)=T4."create", access (0:read/write)=enum16{"read/write", "read-only", "write-only"}."write-only") -> (refnum out=w1186:refnum<file>)  [unwired: 3 in, 2 out]
                        n549 = Bundle("refnum out"=w1164, "refnum out"=w1163) -> (w1162:T6)  [unwired: 1 in]
                        n550 = Send Notification(notification=w1162, notifier=w1188) -> ()  [unwired: 1 in, 2 out]
                        n551 = Write to Text File(file (use dialog)=w1147, text=w1133) -> (refnum out=w1146:refnum<file>)  [unwired: 2 in, 2 out]
                        n552 = Write to Text File(file (use dialog)=w1192, text=w1172) -> (refnum out=w1193:refnum<file>)  [unwired: 2 in, 2 out]
                        n553 = Write to Binary File(file (use dialog)=w1153, data=w1148, 5:FALSE ("prepend array or string size? (T)"), 9:T3."native, host order" ("byte order (0:big-endian, network order)")) -> (refnum out=w1151:refnum<file>)  [unwired: 2 in, 2 out]
                        n554 = Write to Binary File(file (use dialog)=w1186, data=w1184, 5:FALSE ("prepend array or string size? (T)"), 9:T3."native, host order" ("byte order (0:big-endian, network order)")) -> (refnum out=w1176:refnum<file>)  [unwired: 2 in, 2 out]
                        n555 = Close File(refnum=w1146) -> ()  [unwired: 1 in, 2 out]
                        n556 = Close File(refnum=w1193) -> ()  [unwired: 1 in, 2 out]
                        n557 = Close File(refnum=w1151) -> ()  [unwired: 1 in, 2 out]
                        n558 = Close File(refnum=w1176) -> ()  [unwired: 1 in, 2 out]
                      }
                      frame True {
                        n559 = local write "Record"(FALSE ("Record")) -> ()
                        n560 = One Button Dialog(message=w1212) -> ()  [unwired: 1 in, 1 out]
                      }
                    }
                  }
                }
              }
            }
          }
          event "ABEL Stop Button": Value Change {
            # "Stop trapping"
            n561 = event-data() -> ("NewVal"=w1223:bool)  [unwired: 1 in]
            n562 = Join Numbers(hi=u8 1, lo=u8 0) -> ((hi.lo)=w1218:u16)
            n563 = Join Numbers(hi=w1218, lo=u16 0) -> ((hi.lo)=w1221:u32)
            n564 = Build Array(w1221) -> (w1222:u32[])
            n565 = xnode "Invoke Method"("FPGA VI Reference In"=w1216, "Data"=w1222, "Timeout (ms)"=-1) -> ()  [unwired: 1 in, 3 out]
          }
        }
        n566 = feedback-in #14(w364) -> ()
        n567 = feedback-in #15(w362) -> ()
      }
    }
    frame #2 {
      # "Stop resources shared between the loops"
      n568 = xnode "Invoke Method"("FPGA VI Reference In"=w1258) -> ("FPGA VI Reference Out"=w1257:refnum<k20>)  [unwired: 1 in, 1 out]
      n569 = Release Notifier(notifier=w1254) -> ()  [unwired: 2 in, 3 out]
      n570 = Release Notifier(notifier=w1253) -> ()  [unwired: 2 in, 3 out]
      n571 = local write "ABEL Stop Button"(FALSE ("stop")) -> ()
      n572 = local write "Trap"(FALSE ("Trap")) -> ()
      n573 = xnode "Close FPGA VI Reference"("FPGA VI Reference In"=w1257) -> ()  [unwired: 1 in, 1 out]
    }
  }
  n574 = Divide(x=w16, y=w14) -> (x/y=w15:dbl)
  n575 = Divide(x=32767.0 ("Maximum Voltage"), y=3276.8) -> (x/y=w11:dbl)
